vi "ONR Det Tube.vi"() -> ()   [LabVIEW 2018]
uses:
  <vilib>/Utility/file.llb/Write Delimited Spreadsheet (string).vi
  <vilib>/Analysis/NI_AALBase.lvlib
  <vilib>/Analysis/baseanly.llb/Mean (DBL).vi
  <vilib>/Utility/file.llb/Write Delimited Spreadsheet (DBL).vi
panel:
  out "Test row":string[](array[string])
  out "Test CSV Header":string[](array[string])
  out "vac err":dbl caption="Vacuum" format="%.3f %%"
  out "fuel err":dbl caption="Fuel" format="%.3f %%"
  out "ox err":dbl caption="Oxidizer" format="%.3f %%"
  out "dil err":dbl caption="Diluent" format="%.3f %%"
  in  "Vacuum Cutoff":dbl[unit]=689.4757889515781 format="%.2f"
  out "Fuel Cutoff":dbl[unit] caption="Fuel" format="%.2f"
  out "Oxidizer Cutoff":dbl[unit] caption="Oxidizer" format="%.2f"
  out "Diluent Cutoff":dbl[unit] caption="Diluent" format="%.2f"
  out "Test Status":string="No tests loaded"
  in  "Equivalence Ratio":string(combo)
  in  "Diluent":string(combo)
  in  "Diluent Mole Fraction":string(combo)
  in  "Fuel":string(combo)
  in  "Oxidizer":string(combo)
  in  "Initial Pressure":string(combo)
  out "indices":T1
  out "Test CSV":string[][](array[string])
  in  "Purge Time":dbl[unit] format="%#_13g"
  out "Remaining":dbl format="%<%M:%S>t"
  in  "Mix Time":dbl[unit]=180.0 format="%#_13g"
  out "Atmospheric (Calibrated)":dbl[unit]
  out "Diode read complete":bool
  out "Test Over?":bool
  in  "Tube valve delay (ms)":u32=4000
  out "Stop All":bool
  out "Stop Tests":bool
  in  "Pressure sample period (ms)":u32=100
  out "Record Diodes":bool
  out "Pressure Calibration":T2
  out "Pressure\nReadings":T3
  in  "Run Test":bool
  in  "Load Test CSV":bool
  in  "Current State":T4(ring)
  in  "Spark":bool
  in  "Mix Fan":bool
  in  "Stop Valve Control":bool
  in  "Atmospheric Pressure":dbl[unit] format="%.2f"
  in  "Valve Tube Inlet":bool
  in  "Valve Mix Inlet":bool
  in  "Valve Mix Outlet":bool
  in  "Valve Tube Outlet":bool=TRUE
  in  "Valve Oxidizer":bool
  in  "Valve Fuel":bool
  in  "Valve Diluent":bool
  in  "Valve Purge":bool
  in  "Valve Vacuum":bool
  in  "Set Mode":bool=TRUE
  out "Ambient Temp":dbl[unit]=567.411111111111 format="%.2f"
  out "Manifold Temp":dbl[unit]=294.2611111111111 format="%.2f"
  out "Tube Temp":dbl[unit]=294.2611111111111 format="%.2f"
  out "Manifold Pressure":dbl[unit] format="%.2f"
  out "Tube Pressure":dbl[unit] format="%.2f"
  out "System Pressures":T5(graph)={"Fuel Cutoff"=0.0, "Oxidizer Cutoff"=0.0, "Diluent Cutoff"=0.0, "Manifold Pressure"=-7310644.769423339, "Tube Pressure"=114564.88331091503}
  out "Completed fires":i32
  out "Pressure Unsafe?":bool
  # "Set Point"
  # "Error"
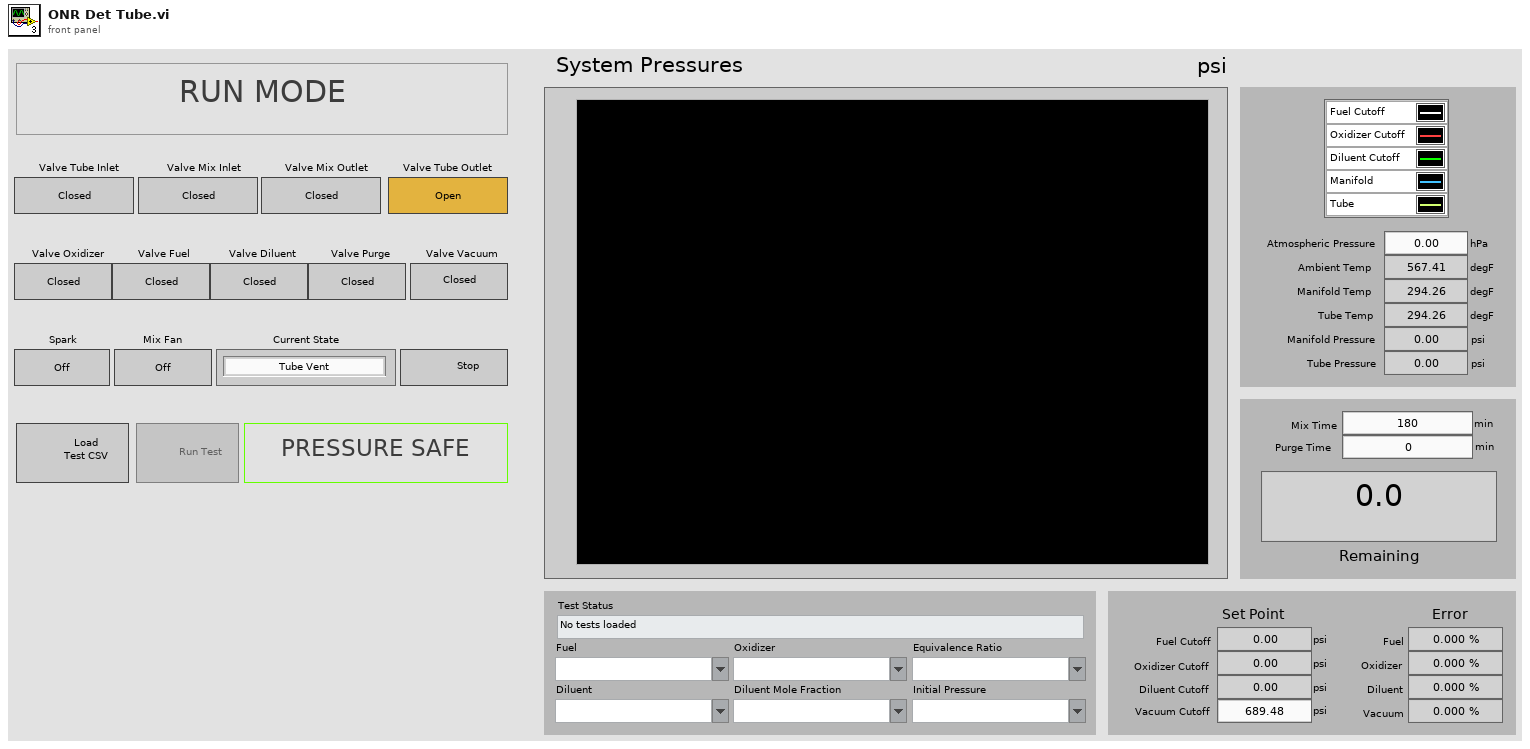
[diagram p1: front panel]
types:
  T1 = cluster{"fuel":i32, "oxidizer":i32, "diluent":i32, "diluent_mol_frac":i32, "equivalence":i32, "init_pressure":i32, "p_f":i32, "p_ox":i32, "p_dil":i32}
  T2 = cluster{"Manifold slope":dbl, "Manifold intercept":dbl, "Tube slope":dbl, "Tube intercept":dbl}
  T3 = cluster{"Time":timestamp, "Tube reading":dbl, "Manifold reading":dbl}
  T4 = enum16{"Tube Vent", "Mix Section Purge", "Tube Purge", "Tube Vacuum", "Diluent Fill", "Oxidizer Fill", "Fuel Fill", "Fill Hold", "Mixing", "Tube Closed", "Ignition", "Manifold Vent"}
  T5 = cluster{"Fuel Cutoff":dbl[unit], "Oxidizer Cutoff":dbl[unit], "Diluent Cutoff":dbl[unit], "Manifold Pressure":dbl[unit], "Tube Pressure":dbl[unit]}
  T6 = enum8{"Enabled", "Disabled", "Disabled and Grayed Out"}
  T7 = enum16{"open", "open or create", "create or replace", "create", "open (read-only)"}
  T8 = cluster{"Fuel Cutoff":dbl[unit], "Oxidizer Cutoff":dbl[unit], "Diluent Cutoff":dbl[unit], "Diluent Cutoff":dbl[unit], "Diluent Cutoff":dbl[unit]}[]
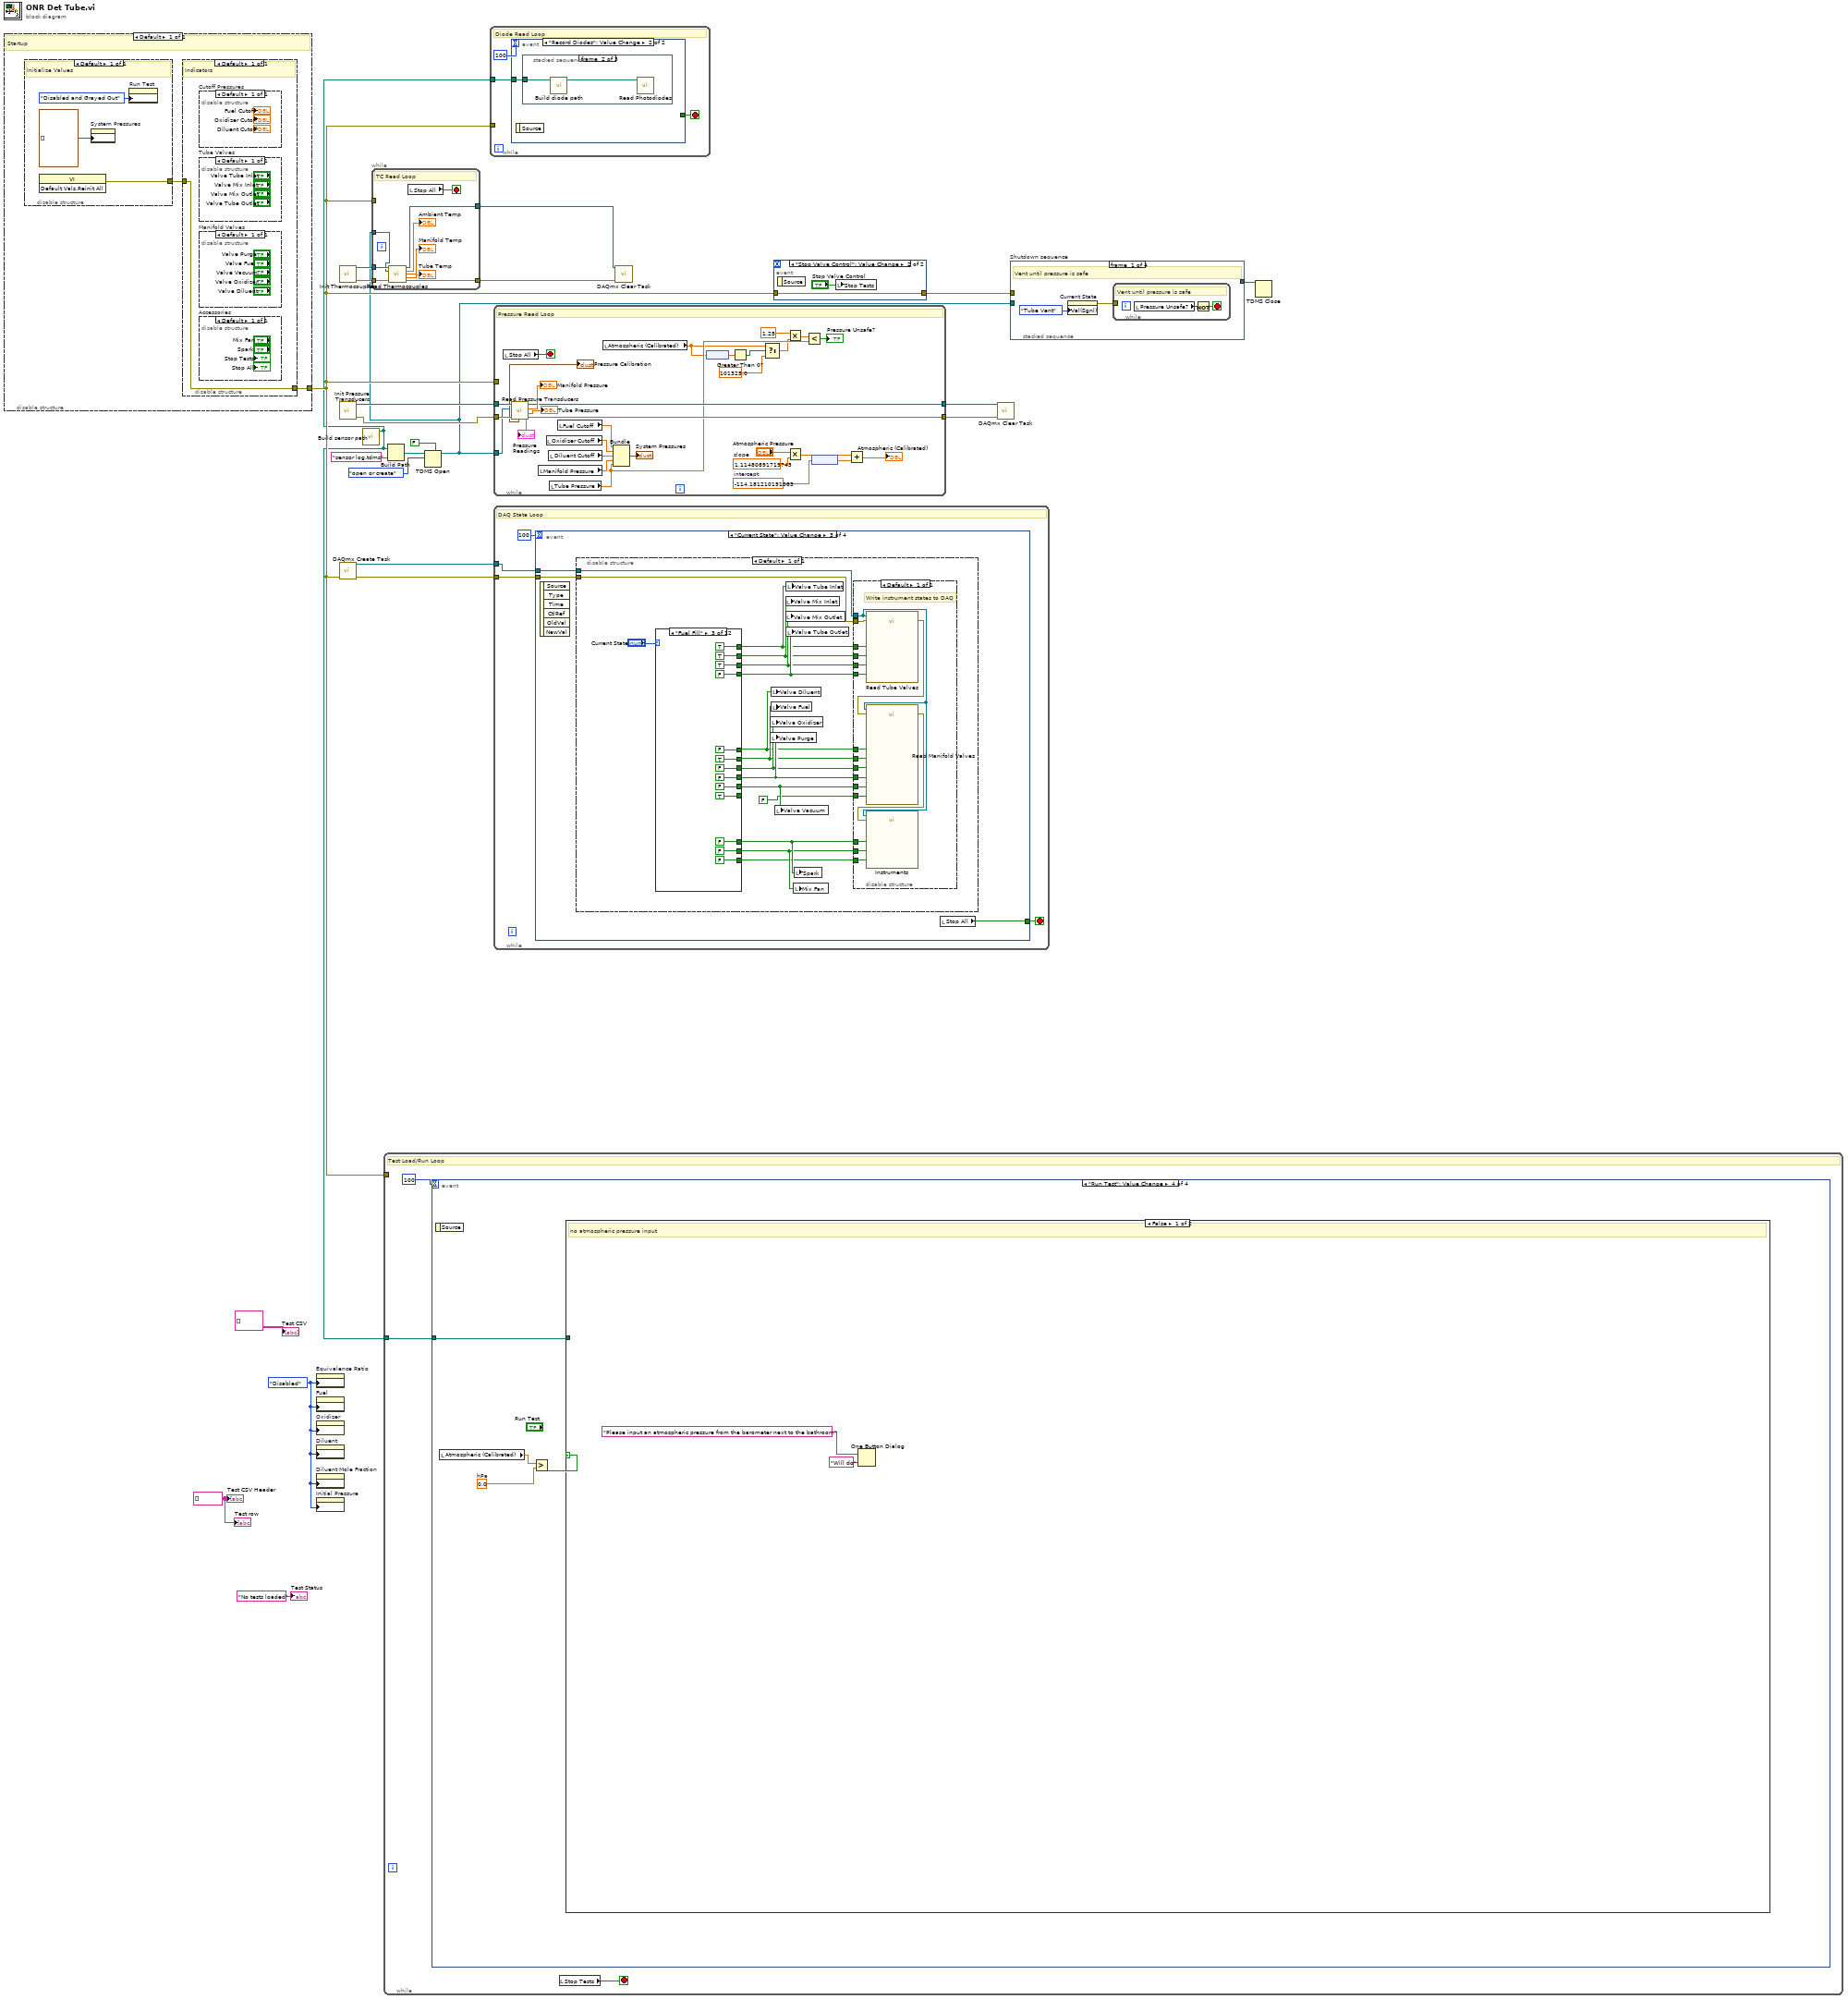
[diagram p0: block diagram]
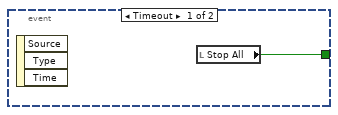
[diagram p2: hidden frame]
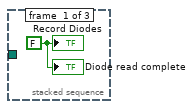
[diagram p3: hidden frame]
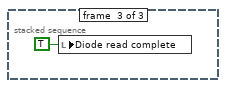
[diagram p4: hidden frame]
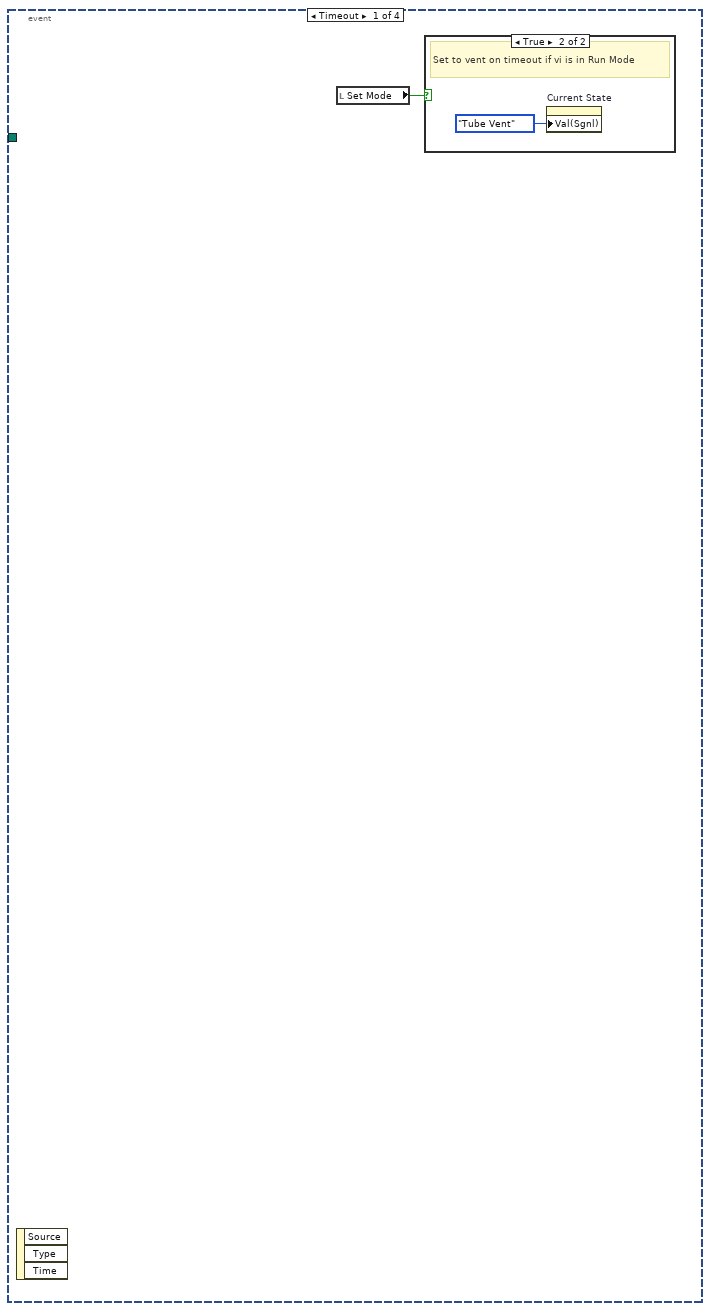
[diagram p5: hidden frame]
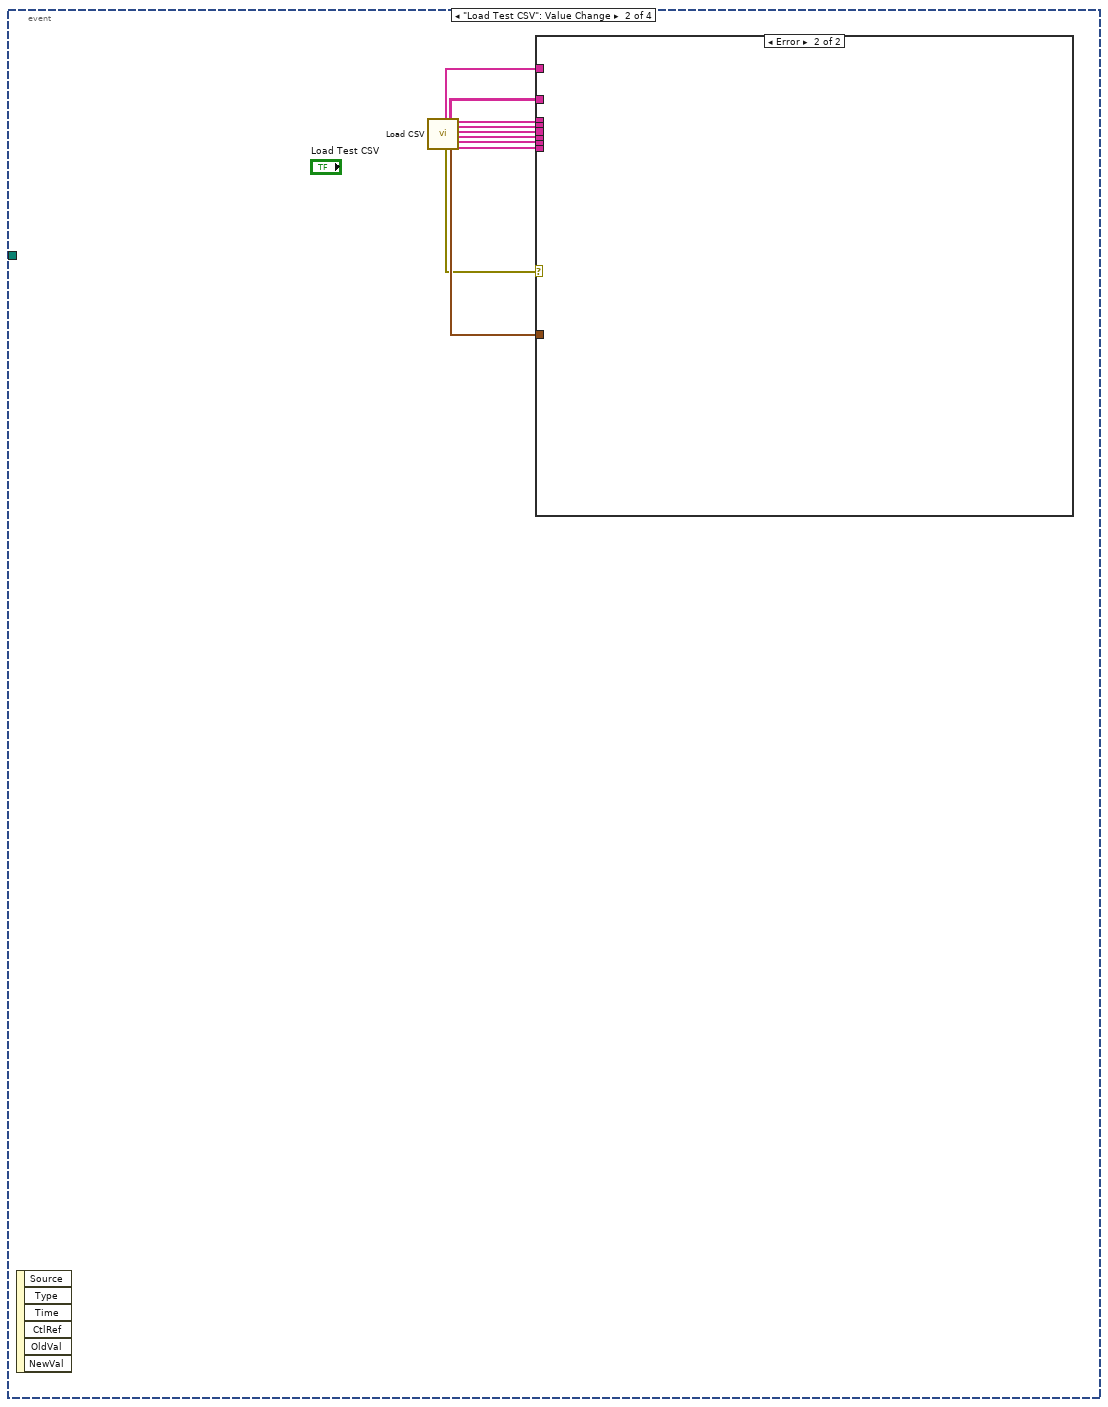
[diagram p7: hidden frame]
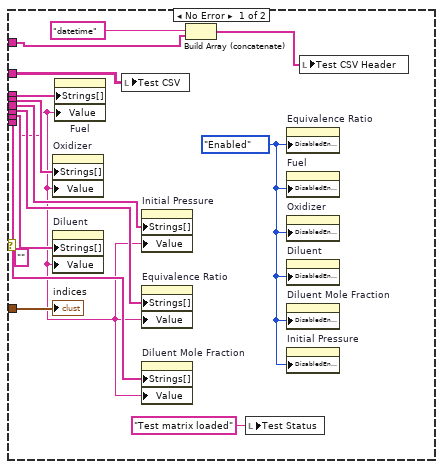
[diagram p8: hidden frame]
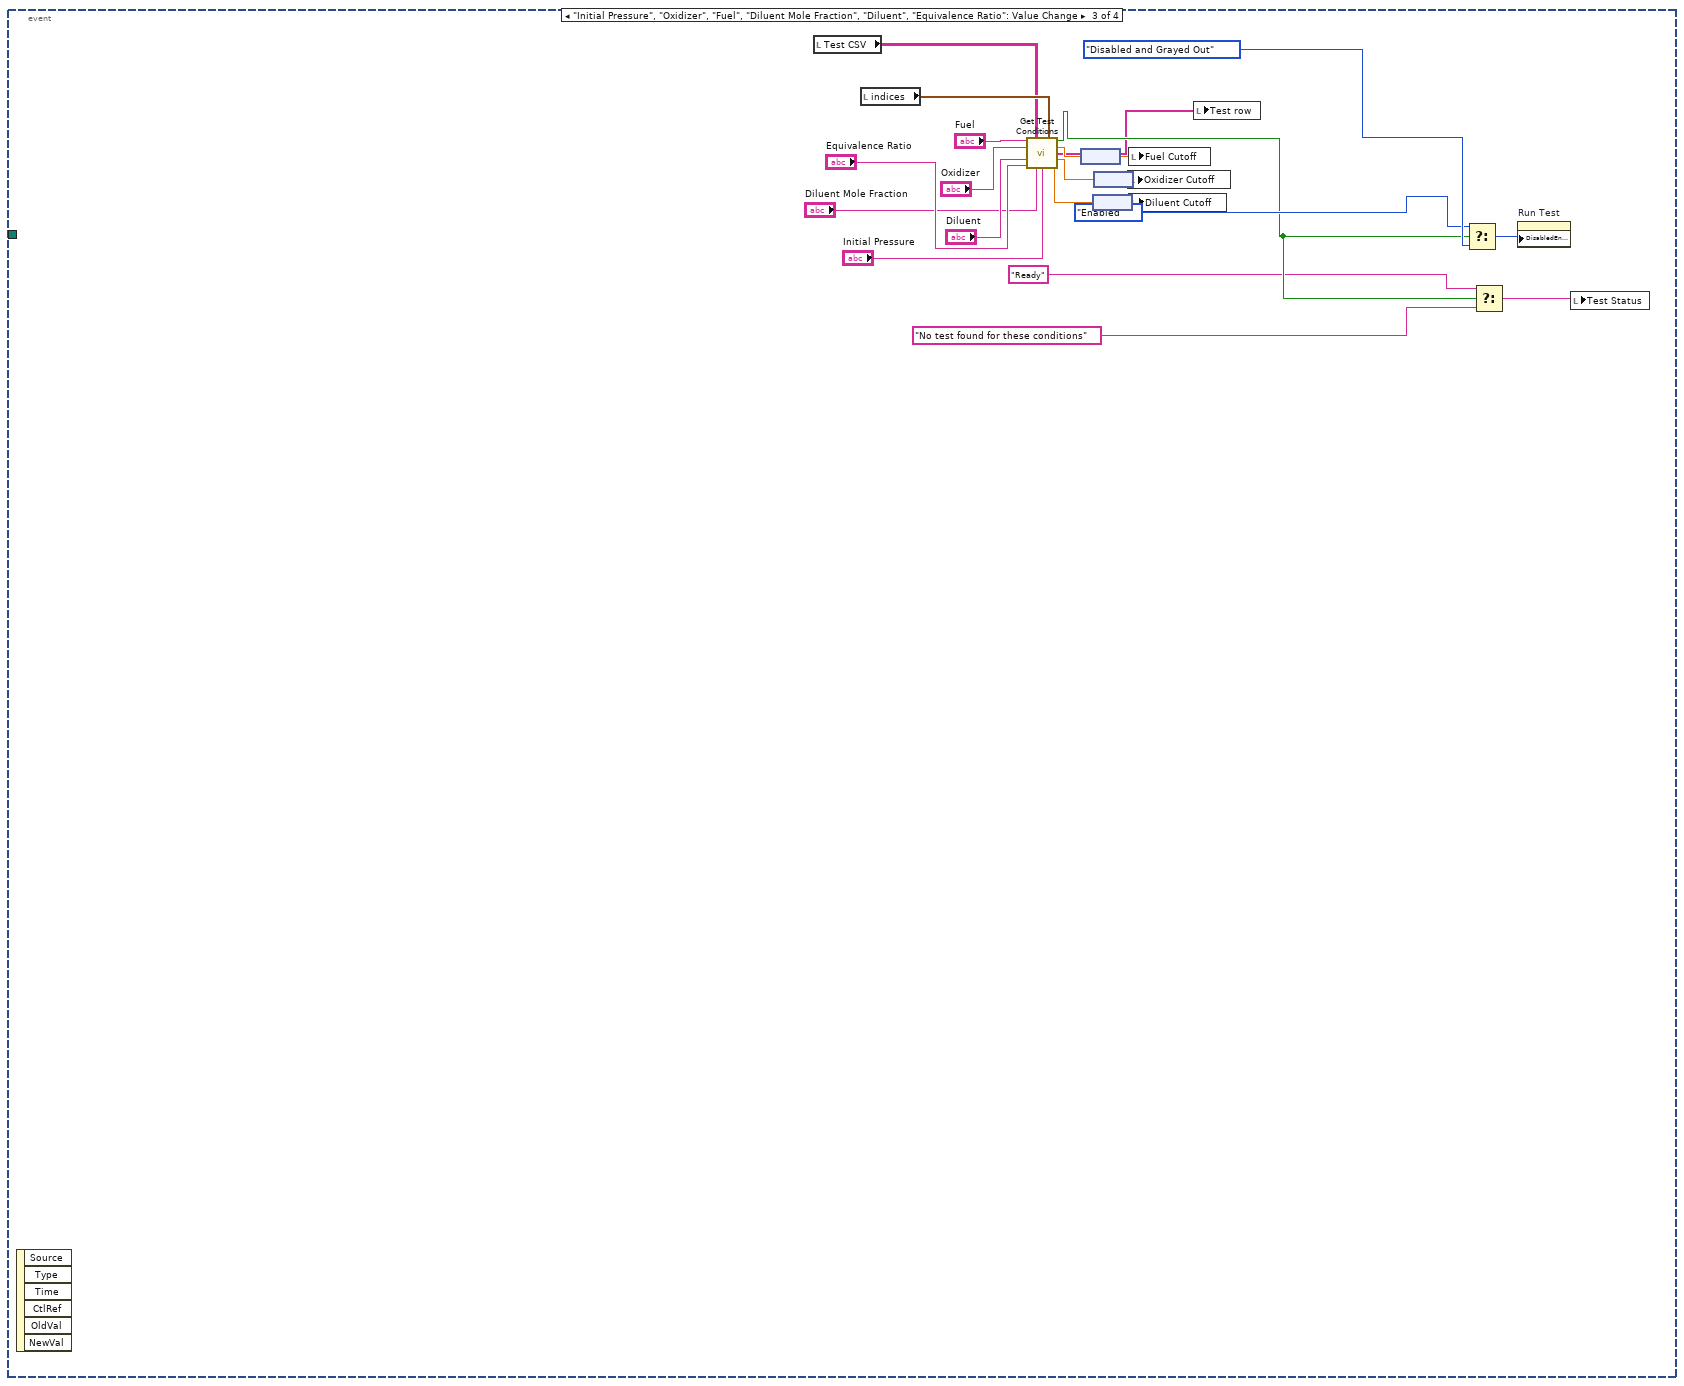
[diagram p9: hidden frame]
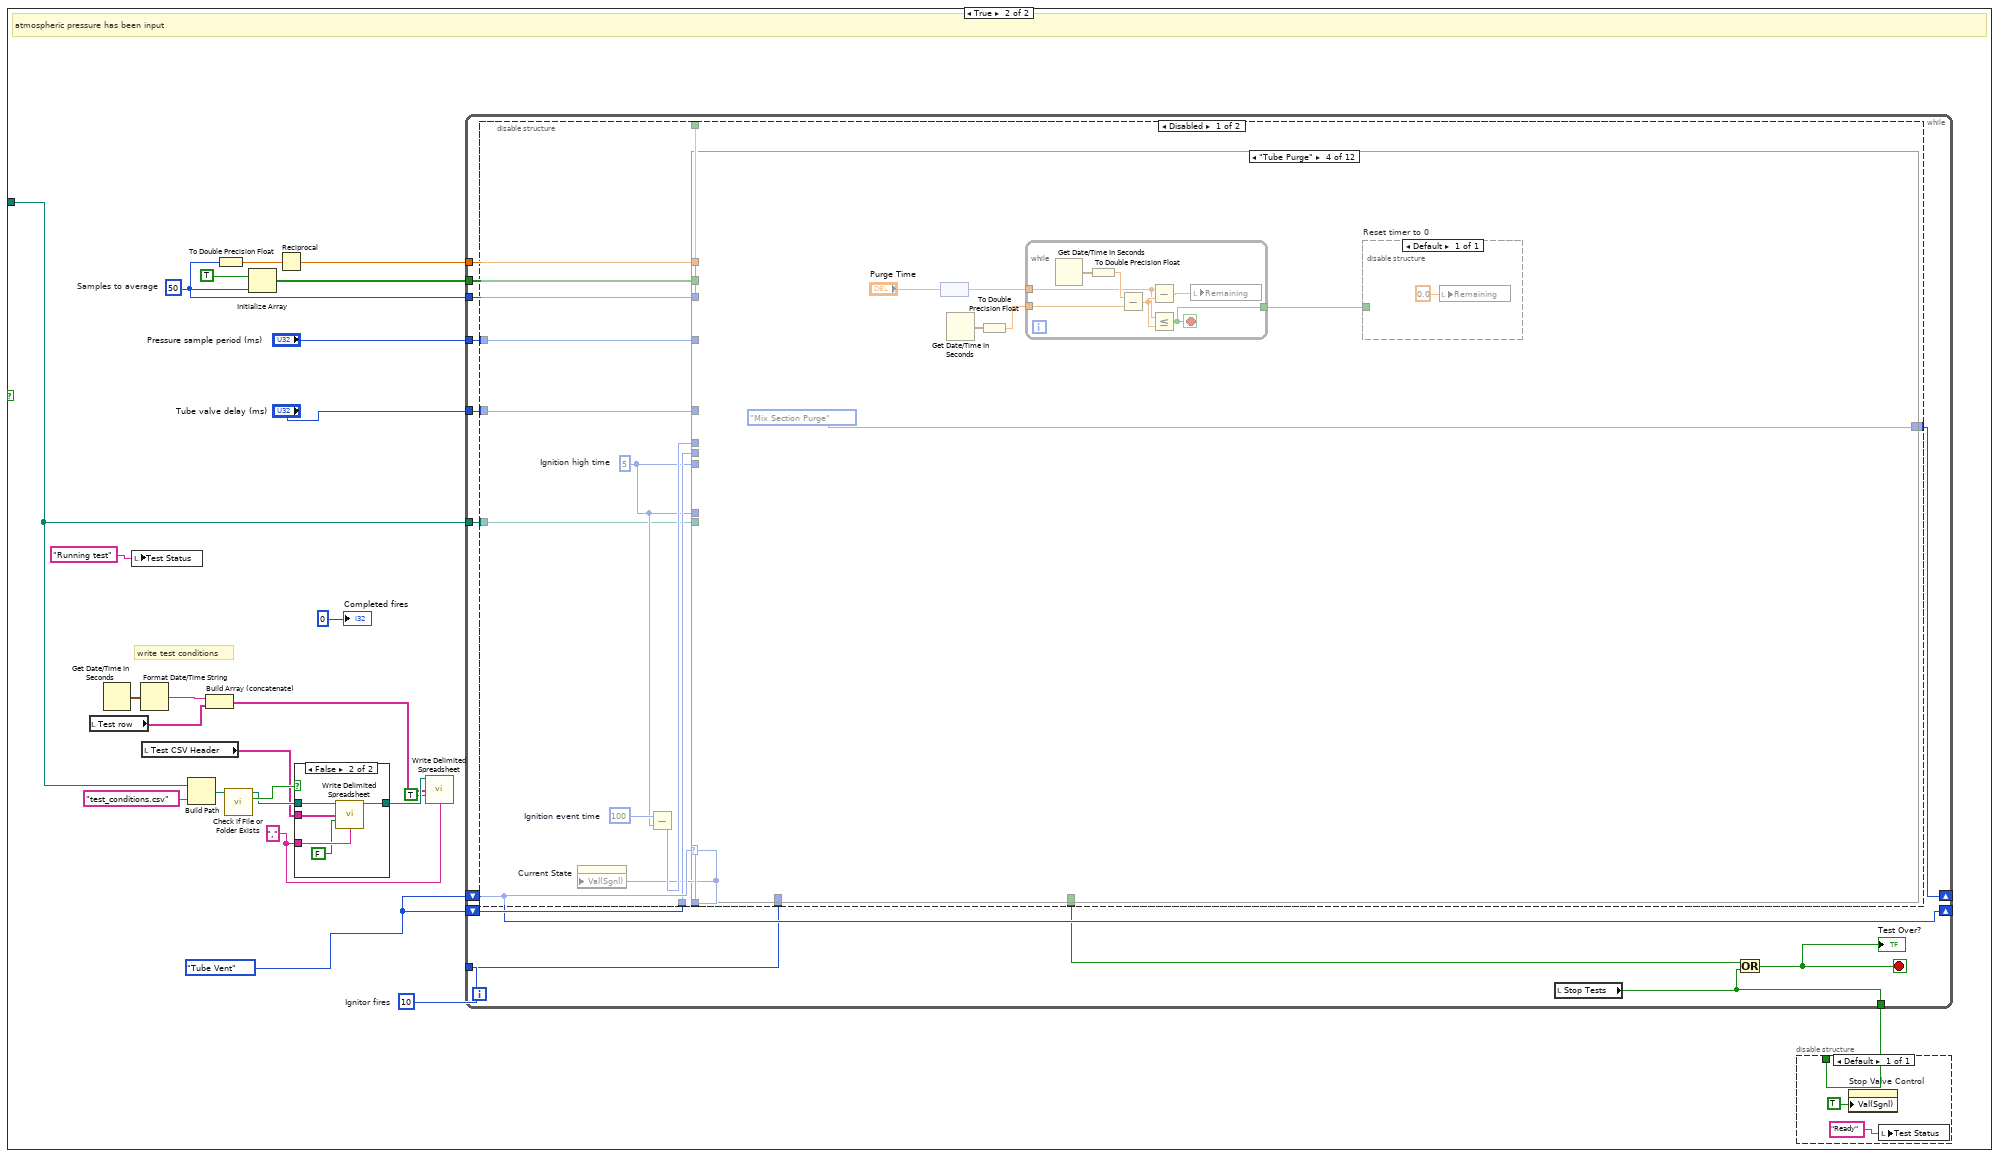
[diagram p10: hidden frame]
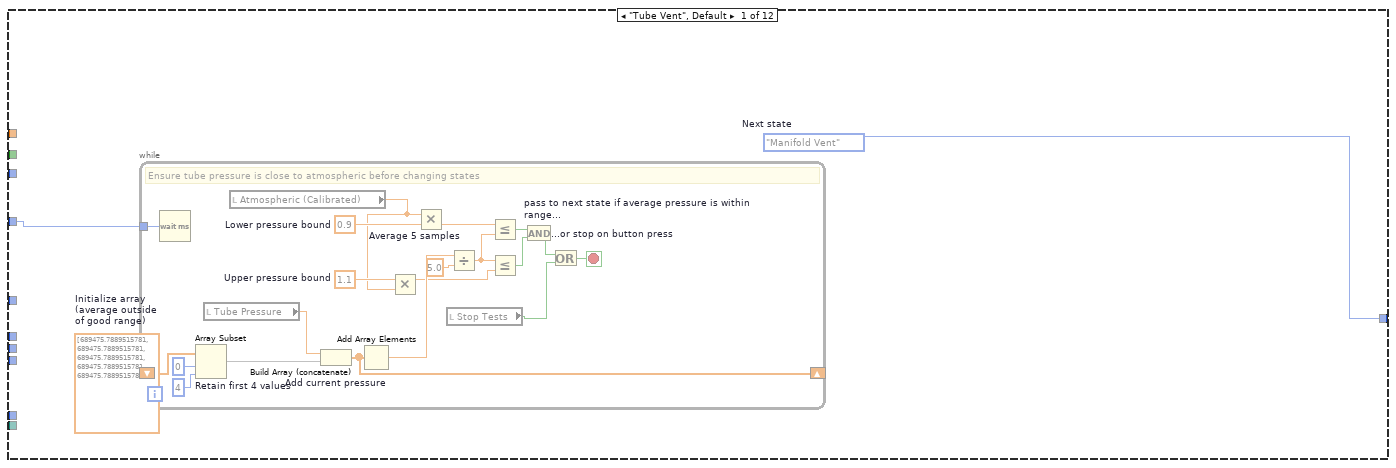
[diagram p12: hidden frame]
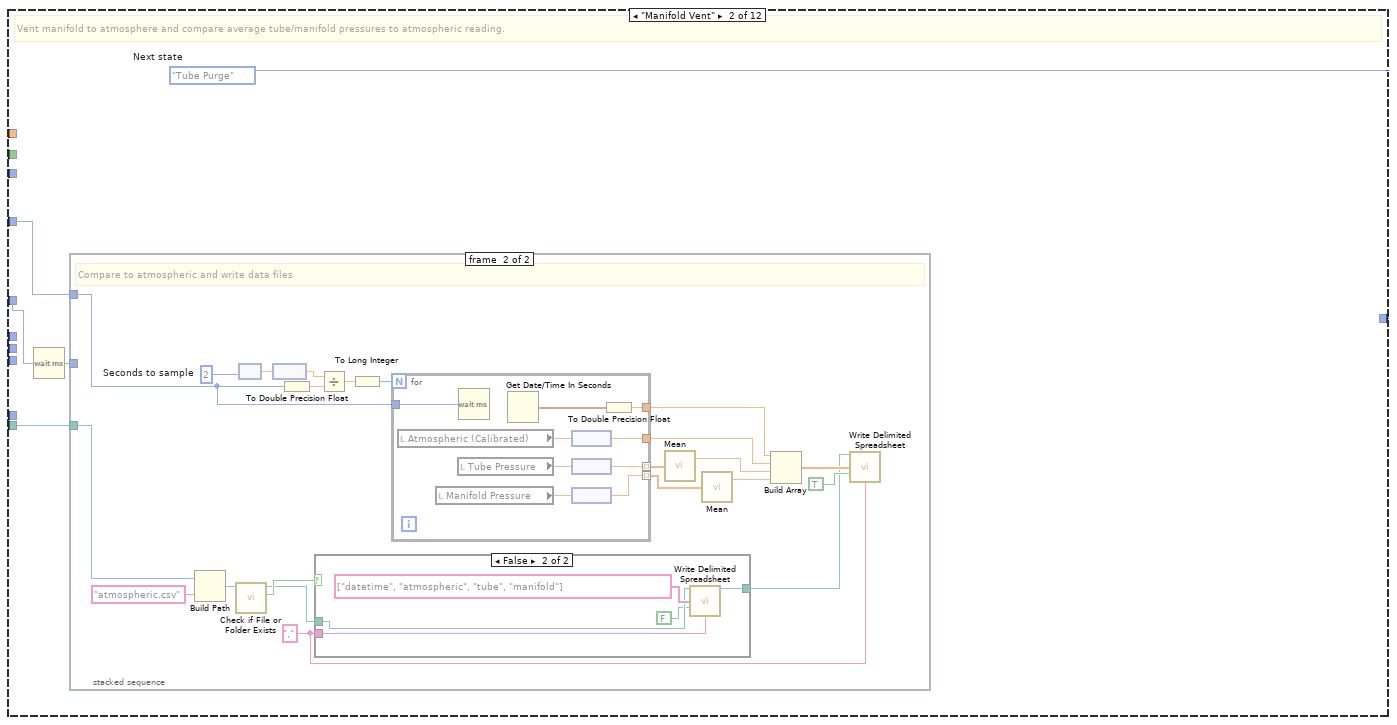
[diagram p13: hidden frame]
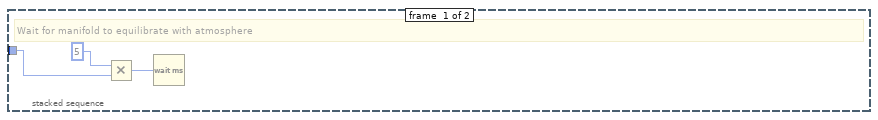
[diagram p14: hidden frame]
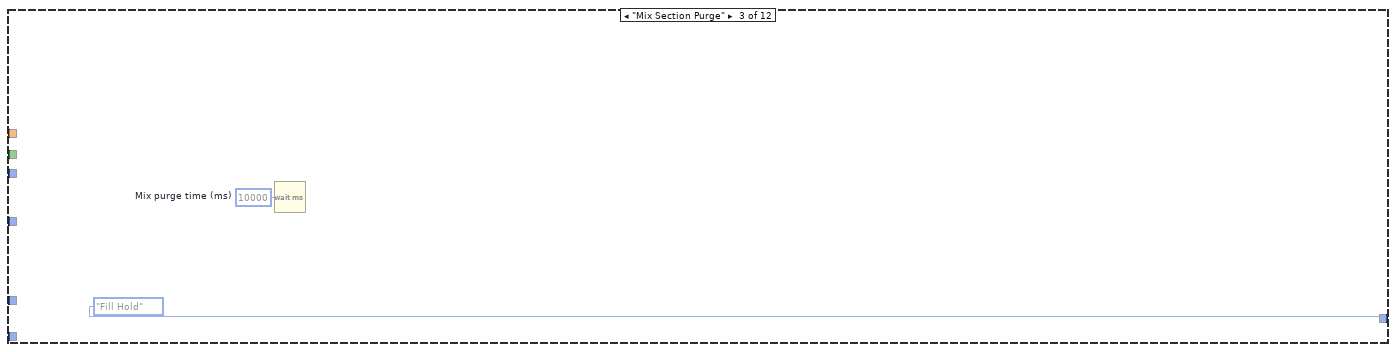
[diagram p16: hidden frame]
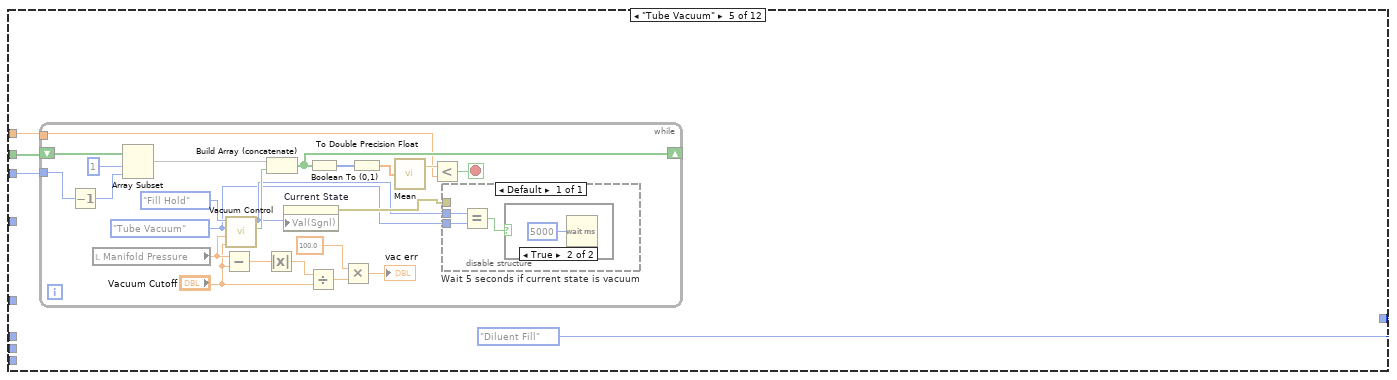
[diagram p17: hidden frame]
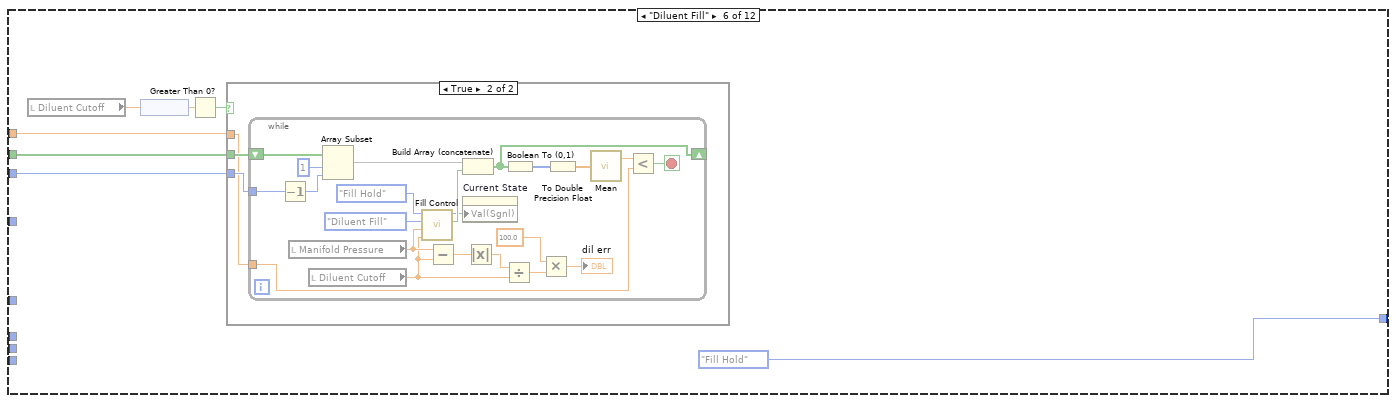
[diagram p19: hidden frame]
diagram:
  w1 = string[] []
  w2 = T6."Disabled" ("Disabled")
  n1 = disable-structure shown="Default" {
    disable-tunnel: [w24] -> w13
    frame Enabled {
      # "Startup"
      n2 = disable-structure shown="Default" {
        disable-tunnel: [w26] -> w25
        frame Enabled {
          # "Initialize Values"
          n3 = invoke class="VI" method="Default Vals.Reinit All"() -> (error out=w26:errorcluster)  [unwired: 3 in, 2 out]
          n4 = property on="System Pressures" class="WFChart (strict)"("History Data"=T8 []) -> ()  [unwired: 2 in, 2 out]
          n5 = property on="Run Test" class="Bool"("DisabledEnum"=T6."Disabled and Grayed Out" ("Disabled")) -> ()  [unwired: 2 in, 2 out]
        }
      }
      n6 = disable-structure shown="Default" {
        disable-tunnel: w25 -> [w29]
        disable-tunnel: [w29] -> w24
        frame Enabled {
          # "Indicators"
          n7 = disable-structure "Cutoff Pressures" shown="Default" {
            frame Enabled {
            }
          }
          n8 = disable-structure "Tube Valves" shown="Default" {
            frame Enabled {
            }
          }
          n9 = disable-structure "Manifold Valves" shown="Default" {
            frame Enabled {
            }
          }
          n10 = disable-structure "Accessories" shown="Default" {
            frame Enabled {
            }
          }
        }
      }
    }
  }
  n11 = property on="Equivalence Ratio" class="CmbBox"("DisabledEnum"=w2) -> ()  [unwired: 2 in, 2 out]
  n12 = property on="Fuel" class="CmbBox"("DisabledEnum"=w2) -> ()  [unwired: 2 in, 2 out]
  n13 = property on="Oxidizer" class="CmbBox"("DisabledEnum"=w2) -> ()  [unwired: 2 in, 2 out]
  n14 = property on="Diluent" class="CmbBox"("DisabledEnum"=w2) -> ()  [unwired: 2 in, 2 out]
  n15 = property on="Diluent Mole Fraction" class="CmbBox"("DisabledEnum"=w2) -> ()  [unwired: 2 in, 2 out]
  n16 = property on="Initial Pressure" class="CmbBox"("DisabledEnum"=w2) -> ()  [unwired: 2 in, 2 out]
  n17 = call "Init Thermocouples.vi"() -> ("task out"=w16:refnum<k21>, "Error Out"=w17:errorcluster)  [unwired: 14 in]
  n18 = call "Init Pressure Transducers.vi"() -> ("Error Out"=w21:errorcluster, "task out"=w20:refnum<k21>)  [unwired: 2 in]
  n19 = call <vilib>:"DAQmx Create Task.vi"("error in"=w13) -> ("task out"=w14:refnum<k21>, "error out"=w15:errorcluster)  [unwired: 13 in]
  n20 = call "Build sensor path.vi"() -> ("Current test directory"=w5:path)  [unwired: 9 in, 1 out]
  n21 = while {
    tunnel: w13 -> [_]
    tunnel: w5 -> [w30]
    stop <- w31 stop-if-true
    # "Test Load/Run Loop"
    n22 = event shown="[3] \"Run Test\": Value Change" {
      selector: _ -> [_ _ _ _]
      dyn-events: _ -> [_ _ _ _]
      timeout: 100 -> [_ _ _ _]
      tunnel: w30 -> [_ _ _ w81]
      event Timeout {
        n23 = event-data() -> ()  [unwired: 1 in, 3 out]
        n24 = local read "Set Mode"() -> (w33:bool)
        n25 = case shown="True" w33 {
          frame False {
          }
          frame True {
            # "Set to vent on timeout if vi is in Run Mode"
            n26 = property on="Current State" class="Enum (strict)"("Val(Sgnl)"=T4."Tube Vent" ("Current State 2")) -> ()  [unwired: 2 in, 2 out]
          }
        }
      }
      event "Load Test CSV": Value Change {
        n27 = event-data() -> ()  [unwired: 1 in, 6 out]
        n28 = call "Load CSV.vi"() -> ("Header"=w35:string[], "error out"=w36:errorcluster, "CSV Array"=w37:string[][], "indices"=w38:T1, "Fuel"=w41:string[], "Oxidizer"=w40:string[], "Initial Pressure"=w39:string[], "Equivalence Ratio"=w42:string[], "Diluent"=w43:string[], "Diluent Mole Fraction"=w44:string[])  [unwired: 10 in]
        n29 = case shown="Error" w36 {
          tunnel: w44 -> [w58 _]
          tunnel: w43 -> [w57 _]
          tunnel: w42 -> [w56 _]
          tunnel: w41 -> [w55 _]
          tunnel: w40 -> [w54 _]
          tunnel: w39 -> [w53 _]
          tunnel: w38 -> [w52 _]
          tunnel: w37 -> [w50 _]
          tunnel: w35 -> [w46 _]
          frame No Error {
            w48 = T6."Enabled" ("Disabled")
            w51 = "" ("Value (Signaling)")
            n30 = property on="Oxidizer" class="CmbBox"("Strings[]"=w54, "Value"=w51) -> ()  [unwired: 2 in, 2 out]
            n31 = property on="Diluent" class="CmbBox"("Strings[]"=w57, "Value"=w51) -> ()  [unwired: 2 in, 2 out]
            n32 = property on="Fuel" class="CmbBox"("Strings[]"=w55, "Value"=w51) -> ()  [unwired: 2 in, 2 out]
            n33 = local write "Test CSV"(w50) -> ()
            n34 = property on="Initial Pressure" class="CmbBox"("Strings[]"=w53, "Value"=w51) -> ()  [unwired: 2 in, 2 out]
            n35 = property on="Equivalence Ratio" class="CmbBox"("Strings[]"=w56, "Value"=w51) -> ()  [unwired: 2 in, 2 out]
            n36 = property on="Diluent Mole Fraction" class="CmbBox"("Strings[]"=w58, "Value"=w51) -> ()  [unwired: 2 in, 2 out]
            n37 = Build Array (concatenate)("datetime", w46) -> (w45:string[])
            n38 = local write "Test Status"("Test matrix loaded" ("Test Status")) -> ()
            n39 = property on="Equivalence Ratio" class="CmbBox"("DisabledEnum"=w48) -> ()  [unwired: 2 in, 2 out]
            n40 = property on="Fuel" class="CmbBox"("DisabledEnum"=w48) -> ()  [unwired: 2 in, 2 out]
            n41 = property on="Oxidizer" class="CmbBox"("DisabledEnum"=w48) -> ()  [unwired: 2 in, 2 out]
            n42 = property on="Diluent" class="CmbBox"("DisabledEnum"=w48) -> ()  [unwired: 2 in, 2 out]
            n43 = property on="Diluent Mole Fraction" class="CmbBox"("DisabledEnum"=w48) -> ()  [unwired: 2 in, 2 out]
            n44 = property on="Initial Pressure" class="CmbBox"("DisabledEnum"=w48) -> ()  [unwired: 2 in, 2 out]
            n45 = local write "Test CSV Header"(w45) -> ()
            "indices" <- w52
          }
          frame Error {
          }
        }
      }
      event "Initial Pressure", "Oxidizer", "Fuel", "Diluent Mole Fraction", "Diluent", "Equivalence Ratio": Value Change {
        n46 = event-data() -> ()  [unwired: 1 in, 6 out]
        n47 = local read "Test CSV"() -> (w67:string[][])
        n48 = local read "indices"() -> (w74:T1)
        n49 = call "Get Test Conditions.vi"("Fuel"="Fuel", "CSV Array"=w67, "indices"=w74, "Oxidizer"="Oxidizer", "Diluent"="Diluent", "Equivalence Ratio"="Equivalence Ratio", "Diluent Mole Fraction"="Diluent Mole Fraction", "Initial Pressure"="Initial Pressure") -> ("Test Found"=w63:bool, "Fuel Partial Pressure"=w73:dbl, "Test row"=w59:string[], "Oxidizer Partial Pressure"=w72:dbl, "Diluent Partial Pressure"=w71:dbl)  [unwired: 3 in]
        n50 = node(w73) -> (w70:dbl[unit])
        n51 = node(w71) -> (w68:dbl[unit])
        n52 = node(w72) -> (w69:dbl[unit])
        n53 = local write "Oxidizer Cutoff"(w69) -> ()
        n54 = local write "Fuel Cutoff"(w70) -> ()
        n55 = local write "Diluent Cutoff"(w68) -> ()
        n56 = local write "Test row"(w59) -> ()
        n57 = Select(t=T6."Enabled" ("Disabled"), s=w63, f=T6."Disabled and Grayed Out" ("Disabled")) -> (s? t:f=w66:T6)
        n58 = Select(t="Ready", s=w63, f="No test found for these conditions") -> (s? t:f=w62:string)
        n59 = property on="Run Test" class="Bool"("DisabledEnum"=w66) -> ()  [unwired: 2 in, 2 out]
        n60 = local write "Test Status"(w62) -> ()
      }
      event "Run Test": Value Change {
        w83 = dbl[unit] 0.0  # hPa
        n61 = event-data() -> ()  [unwired: 1 in, 1 out]
        n62 = local read "Atmospheric (Calibrated)"() -> (w84:dbl[unit])
        n63 = Greater?(x=w84, y=w83) -> (0:w82:bool)
        n64 = case shown="False" w82 {
          tunnel: w81 -> [_ w93]
          frame False {
            # "no atmospheric pressure input"
            n65 = One Button Dialog(message="Please input an atmospheric pressure from the barometer next to the bathroom" ("source"), button name ("OK")="Will do") -> ()  [unwired: 1 out]
          }
          frame True {
            w88 = "," ("delimiter (\\t)")
            w102 = 10  # Ignitor fires
            w104 = 50  # Samples to average
            w106 = T4."Tube Vent" ("Current State 2")
            # "write test conditions"
            # "atmospheric pressure has been input"
            n66 = local read "Test row"() -> (w90:string[])
            n67 = Get Date/Time In Seconds() -> (seconds since 1Jan1904=w99:timestamp)
            n68 = local write "Test Status"("Running test" ("Test Status")) -> ()
            n69 = Format Date/Time String(seconds (now)=w99) -> (date/time string=w98:string)  [unwired: 2 in]
            n70 = local read "Test CSV Header"() -> (w92:string[])
            n71 = Build Path(base path=w93, name or relative path="test_conditions.csv") -> (appended path=w95:path)
            n72 = Build Array (concatenate)(w98, w90) -> (w89:string[])
            n73 = To Double Precision Float(number=w104) -> (double precision float=w107:dbl)
            n74 = call <vilib>:"Check if File or Folder Exists.vi"("path"=w95) -> ("file or folder exists?"=w97:bool, "dup path"=w96:path)  [unwired: 8 in, 1 out]
            n75 = Initialize Array(TRUE, w104) -> (w109:bool[])
            n76 = Reciprocal(x=w107) -> (1/x=w110:dbl)
            n77 = case shown="False" w97 {
              tunnel: w88 -> [_ w117]
              tunnel: [w112 w116] -> w91
              tunnel: w96 -> [w112 w115]
              tunnel: w92 -> [_ w113]
              frame True {
              }
              frame False {
                n78 = call-poly <vilib>:"Write Delimited Spreadsheet.vi"("file path (dialog if empty)"=w115, "1D data"=w113, "append to file? (new file:F)"=FALSE, "delimiter (\\t)"=w117) -> ("new file path (Not A Path if cancelled)"=w116:path)  [unwired: 10 in, 1 out]
              }
            }
            n79 = call-poly <vilib>:"Write Delimited Spreadsheet.vi"("file path (dialog if empty)"=w91, "1D data"=w89, "append to file? (new file:F)"=TRUE, "delimiter (\\t)"=w88) -> ()  [unwired: 10 in, 2 out]
            n80 = while {
              shift-right: [w130] -> _
              shift-left: w106 -> [w123]
              shift-right: [w123] -> _
              shift-left: w106 -> [w129]
              tunnel: "Tube valve delay (ms)" -> [w127]
              tunnel: w109 -> [w124]
              tunnel: w104 -> [w125]
              tunnel: w110 -> [w126]
              tunnel: "Pressure sample period (ms)" -> [w128]
              tunnel: [w121] -> w103
              tunnel: w102 -> [w122]
              tunnel: w93 -> [w118]
              stop <- w120 stop-if-true
              n81 = disable-structure shown="Disabled" {
                disable-tunnel: [w144 _] -> w130
                disable-tunnel: w129 -> [w143 _]
                disable-tunnel: w128 -> [w142 _]
                disable-tunnel: w127 -> [w141 _]
                disable-tunnel: w126 -> [w140 _]
                disable-tunnel: w125 -> [w139 _]
                disable-tunnel: w124 -> [w138 _]
                disable-tunnel: w123 -> [w135 _]
                disable-tunnel: w122 -> [w134 _]
                disable-tunnel: [w133 _] -> w119
                disable-tunnel: w118 -> [w131 _]
                frame Disabled {
                  w137 = u32 100  # Ignition event time
                  w132 = u32 5  # Ignition high time
                  n82 = property on="Current State" class="Enum (strict)"("Val(Sgnl)"=w135) -> ()  [unwired: 2 in, 2 out]
                  n83 = Subtract(x=w137, y=w132) -> (x-y=w136:u32)
                  n84 = case shown="\"Tube Purge\"" w135 {
                    tunnel: [w147 w172 T4."Fill Hold" ("Current State 2") T4."Mix Section Purge" ("Current State 2") T4."Diluent Fill" ("Current State 2") T4."Fill Hold" ("Current State 2") T4."Fill Hold" ("Current State 2") T4."Fill Hold" ("Current State 2") w347 T4."Tube Closed" ("Current State 2") w378 T4."Tube Closed" ("Current State 2")] -> w144
                    tunnel: w143 -> [_ _ _ _ _ _ _ _ w348 _ w379 _]
                    tunnel: w142 -> [w146 w171 _ _ _ _ _ _ _ _ _ _]
                    tunnel: w141 -> [_ w170 _ _ _ _ _ _ w345 _ w376 _]
                    tunnel: w140 -> [_ _ _ _ w231 w261 w293 w320 _ _ _ _]
                    tunnel: w139 -> [_ _ _ _ w229 w263 w294 w319 _ _ _ _]
                    tunnel: w138 -> [_ _ _ _ w230 w262 w292 w318 _ _ _ _]
                    tunnel: w132 -> [_ _ _ _ _ _ _ _ _ _ _ _]
                    tunnel: w136 -> [_ _ _ _ _ _ _ _ _ _ w377 _]
                    tunnel: w134 -> [_ _ _ _ _ _ _ _ _ _ w375 _]
                    tunnel: [_ _ _ _ _ _ _ _ _ _ w374 _] -> w133
                    tunnel: w132 -> [_ _ _ _ _ _ _ _ _ _ _ w424]
                    tunnel: w131 -> [_ w168 _ _ _ _ _ _ _ _ w373 _]
                    frame "Tube Vent", Default {
                      w145 = dbl[unit][] [689475.7889515781, 689475.7889515781, 689475.7889515781, 689475.7889515781, 689475.7889515781]  # Initialize array (average outside of good range)
                      w147 = T4."Manifold Vent"  # Next state
                      n85 = while {
                        shift-right: [w166] -> _
                        shift-left: w145 -> [w165]
                        tunnel: w146 -> [w154]
                        stop <- w153 stop-if-true
                        w155 = 0.9  # Lower pressure bound
                        w159 = 1.1  # Upper pressure bound
                        # "Ensure tube pressure is close to atmospheric before changing states"
                        n86 = Wait (ms)(milliseconds to wait=w154) -> ()  [unwired: 1 out]
                        n87 = Array Subset "Retain first 4 values"(array=w165, index=0, length=4) -> (w161:dbl[unit][])
                        n88 = local read "Tube Pressure"() -> (w160:dbl[unit])
                        n89 = local read "Atmospheric (Calibrated)"() -> (w149:dbl[unit])
                        n90 = Build Array (concatenate) "Add current pressure"(w160, w161) -> (w166:dbl[unit][])
                        n91 = Add Array Elements(numeric array=w166) -> (sum=w167:dbl[unit])
                        n92 = Multiply(x=w159, y=w149) -> (x*y=w150:dbl[unit])
                        n93 = Multiply(x=w149, y=w155) -> (x*y=w151:dbl[unit])
                        n94 = local read "Stop Tests"() -> (w148:bool)
                        n95 = Divide "Average 5 samples"(x=w167, y=5.0 ("length")) -> (x/y=w156:dbl[unit])
                        n96 = Less Or Equal?(x=w151, y=w156) -> (x <= y?=w157:bool)
                        n97 = Less Or Equal?(x=w156, y=w150) -> (x <= y?=w158:bool)
                        n98 = And "pass to next state if average pressure is within range..."(x=w157, y=w158) -> (x .and. y?=w152:bool)
                        n99 = Or "...or stop on button press"(x=w152, y=w148) -> (x .or. y?=w153:bool)
                      }
                    }
                    frame "Manifold Vent" {
                      w172 = T4."Tube Purge"  # Next state
                      # "Vent manifold to atmosphere and compare average tube/manifold pressures to atmospheric reading."
                      n100 = Wait (ms)(milliseconds to wait=w170) -> (millisecond timer value=w169:u32)
                      n101 = stacked-sequence {
                        tunnel: w171 -> [w174 w197]
                        tunnel: w169 -> [_ _]
                        tunnel: w168 -> [_ w178]
                        frame #0 {
                          # "Wait for manifold to equilibrate with atmosphere"
                          n102 = Multiply(x=u32 5, y=w174) -> (x*y=w173:u32)
                          n103 = Wait (ms)(milliseconds to wait=w173) -> ()  [unwired: 1 out]
                        }
                        frame #1 {
                          w176 = "," ("delimiter (\\t)")
                          w195 = 2  # Seconds to sample
                          # "Compare to atmospheric and write data files"
                          n104 = Build Path(base path=w178, name or relative path="atmospheric.csv") -> (appended path=w180:path)
                          n105 = call <vilib>:"Check if File or Folder Exists.vi"("path"=w180) -> ("file or folder exists?"=w182:bool, "dup path"=w181:path)  [unwired: 8 in, 1 out]
                          n106 = node(w195) -> (w196:dbl[unit])
                          n107 = node(w196) -> (w194:dbl)
                          n108 = To Double Precision Float(number=w197) -> (double precision float=w191:dbl)
                          n109 = case shown="False" w182 {
                            tunnel: w176 -> [_ w203]
                            tunnel: [w198 w202] -> w183
                            tunnel: w181 -> [w198 w200]
                            frame True {
                            }
                            frame False {
                              n110 = call-poly <vilib>:"Write Delimited Spreadsheet.vi"("file path (dialog if empty)"=w200, "1D data"=string[] ["datetime", "atmospheric", "tube", "manifold"], "append to file? (new file:F)"=FALSE, "delimiter (\\t)"=w203) -> ("new file path (Not A Path if cancelled)"=w202:path)  [unwired: 10 in, 1 out]
                            }
                          }
                          n111 = Divide(x=w194, y=w191) -> (x/y=w193:dbl)
                          n112 = To Long Integer(number=w193) -> (32bit integer=w192:i32)
                          n113 = for {
                            N: w192 -> [_]
                            tunnel: w197 -> [w206]
                            tunnel: [w207] -> w189 mode=indexing
                            tunnel: [w208] -> w190 mode=indexing
                            tunnel: [w209] -> w186
                            tunnel: [w204] -> w177
                            n114 = local read "Atmospheric (Calibrated)"() -> (w210:dbl[unit])
                            n115 = local read "Manifold Pressure"() -> (w212:dbl[unit])
                            n116 = local read "Tube Pressure"() -> (w211:dbl[unit])
                            n117 = Wait (ms)(milliseconds to wait=w206) -> ()  [unwired: 1 out]
                            n118 = Get Date/Time In Seconds() -> (seconds since 1Jan1904=w205:timestamp)
                            n119 = node(w210) -> (w209:dbl)
                            n120 = node(w211) -> (w208:dbl)
                            n121 = node(w212) -> (w207:dbl)
                            n122 = To Double Precision Float(number=w205) -> (double precision float=w204:dbl)
                          }
                          n123 = call-poly <vilib>:"Mean.vi"("X"=w190) -> ("mean"=w187:dbl)  [unwired: 1 out]
                          n124 = call-poly <vilib>:"Mean.vi"("X"=w189) -> ("mean"=w188:dbl)  [unwired: 1 out]
                          n125 = Build Array(w177, w186, w187, w188) -> (w184:dbl[])
                          n126 = call-poly <vilib>:"Write Delimited Spreadsheet.vi"("file path (dialog if empty)"=w183, "1D data"=w184, "append to file? (new file:F)"=TRUE, "delimiter (\\t)"=w176) -> ()  [unwired: 10 in, 2 out]
                        }
                      }
                    }
                    frame "Mix Section Purge" {
                      w213 = u32 10000  # Mix purge time (ms)
                      n127 = Wait (ms)(milliseconds to wait=w213) -> ()  [unwired: 1 out]
                    }
                    frame "Tube Purge" {
                      n128 = node("Purge Time") -> (w215:dbl)
                      n129 = Get Date/Time In Seconds() -> (seconds since 1Jan1904=w218:timestamp)
                      n130 = To Double Precision Float(number=w218) -> (double precision float=w217:dbl)
                      n131 = while {
                        tunnel: w217 -> [w227]
                        tunnel: w215 -> [w224]
                        tunnel: [w223] -> w216
                        stop <- w223 stop-if-true
                        n132 = Get Date/Time In Seconds() -> (seconds since 1Jan1904=w228:timestamp)
                        n133 = To Double Precision Float(number=w228) -> (double precision float=w226:dbl)
                        n134 = Subtract(x=w226, y=w227) -> (x-y=w225:dbl)
                        n135 = Subtract(x=w224, y=w225) -> (x-y=w222:dbl)
                        n136 = Less Or Equal?(x=w224, y=w225) -> (x <= y?=w223:bool)
                        n137 = local write "Remaining"(w222) -> ()
                      }
                      n138 = disable-structure "Reset timer to 0" shown="Default" {
                        disable-tunnel: w216 -> [_]
                        frame Enabled {
                          n139 = local write "Remaining"(0.0 ("Remaining")) -> ()
                        }
                      }
                    }
                    frame "Tube Vacuum" {
                      n140 = while {
                        tunnel: w229 -> [w253]
                        shift-right: [w246] -> _
                        shift-left: w230 -> [w252]
                        tunnel: w231 -> [w245]
                        stop <- w244 stop-if-true
                        w233 = T4."Tube Vacuum" ("Current State 2")
                        n141 = Decrement(x=w253) -> (x-1=w255:i32)
                        n142 = local read "Manifold Pressure"() -> (w241:dbl[unit])
                        n143 = Array Subset(array=w252, index=1, length=w255) -> (w248:bool[])
                        n144 = Subtract(x=w241, y="Vacuum Cutoff") -> (x-y=w242:dbl[unit])
                        n145 = call "Vacuum Control.vi"("Fill Cutoff Pressure"="Vacuum Cutoff", "Manifold Pressure"=w241, "Fill State"=w233, "Hold State"=T4."Fill Hold" ("Current State 2")) -> ("Valve Open?"=w247:bool, "Output State"=w235:T4)  [unwired: 6 in]
                        n146 = Absolute Value(x=w242) -> (abs(x)=w243:dbl[unit])
                        n147 = Build Array (concatenate)(w248, w247) -> (w246:bool[])
                        n148 = property on="Current State" class="Enum (strict)"("Val(Sgnl)"=w235) -> (error out=w236:errorcluster)  [unwired: 2 in, 1 out]
                        n149 = Divide(x=w243, y="Vacuum Cutoff") -> (x/y=w240:dbl)
                        n150 = Boolean To (0,1)(Boolean=w246) -> (0, 1=w249:i16[])
                        n151 = Multiply(x=100.0, y=w240) -> (x*y=→"vac err":dbl)
                        n152 = To Double Precision Float(number=w249) -> (double precision float=w250:dbl[])
                        n153 = call-poly <vilib>:"Mean.vi"("X"=w250) -> ("mean"=w251:dbl)  [unwired: 1 out]
                        n154 = Less?(x=w251, y=w245) -> (x < y?=w244:bool)
                        n155 = disable-structure "Wait 5 seconds if current state is vacuum" shown="Default" {
                          disable-tunnel: w236 -> [_]
                          disable-tunnel: w235 -> [w257]
                          disable-tunnel: w233 -> [w256]
                          frame Enabled {
                            n156 = Equal?(x=w257, y=w256) -> (x = y?=w258:bool)
                            n157 = case shown="True" w258 {
                              frame False {
                              }
                              frame True {
                                n158 = Wait (ms)(milliseconds to wait=u32 5000) -> ()  [unwired: 1 out]
                              }
                            }
                          }
                        }
                      }
                    }
                    frame "Diluent Fill" {
                      n159 = local read "Diluent Cutoff"() -> (w264:dbl[unit])
                      n160 = node(w264) -> (w260:dbl)
                      n161 = Greater Than 0?(x=w260) -> (x > 0?=w265:bool)
                      n162 = case shown="True" w265 {
                        tunnel: w262 -> [_ w269]
                        tunnel: w263 -> [_ w268]
                        tunnel: w261 -> [_ w267]
                        frame False {
                        }
                        frame True {
                          n163 = while {
                            tunnel: w268 -> [w289]
                            shift-right: [w282] -> _
                            shift-left: w269 -> [w288]
                            tunnel: w267 -> [w281]
                            stop <- w280 stop-if-true
                            n164 = Decrement(x=w289) -> (x-1=w291:i32)
                            n165 = local read "Manifold Pressure"() -> (w277:dbl[unit])
                            n166 = local read "Diluent Cutoff"() -> (w276:dbl[unit])
                            n167 = Array Subset(array=w288, index=1, length=w291) -> (w284:bool[])
                            n168 = call "Fill Control.vi"("Fill Cutoff Pressure"=w276, "Manifold Pressure"=w277, "Fill State"=T4."Diluent Fill" ("Current State 2"), "Hold State"=T4."Fill Hold" ("Current State 2")) -> ("Valve Open?"=w283:bool, "Output State"=w273:T4)  [unwired: 6 in]
                            n169 = Subtract(x=w277, y=w276) -> (x-y=w278:dbl[unit])
                            n170 = Build Array (concatenate)(w284, w283) -> (w282:bool[])
                            n171 = property on="Current State" class="Enum (strict)"("Val(Sgnl)"=w273) -> ()  [unwired: 2 in, 2 out]
                            n172 = Absolute Value(x=w278) -> (abs(x)=w279:dbl[unit])
                            n173 = Divide(x=w279, y=w276) -> (x/y=w272:dbl)
                            n174 = Boolean To (0,1)(Boolean=w282) -> (0, 1=w285:i16[])
                            n175 = Multiply(x=100.0, y=w272) -> (x*y=→"dil err":dbl)
                            n176 = To Double Precision Float(number=w285) -> (double precision float=w286:dbl[])
                            n177 = call-poly <vilib>:"Mean.vi"("X"=w286) -> ("mean"=w287:dbl)  [unwired: 1 out]
                            n178 = Less?(x=w287, y=w281) -> (x < y?=w280:bool)
                          }
                        }
                      }
                    }
                    frame "Oxidizer Fill" {
                      n179 = while {
                        tunnel: w294 -> [w315]
                        shift-right: [w308] -> _
                        shift-left: w292 -> [w314]
                        tunnel: w293 -> [w307]
                        stop <- w306 stop-if-true
                        n180 = Decrement(x=w315) -> (x-1=w317:i32)
                        n181 = local read "Manifold Pressure"() -> (w303:dbl[unit])
                        n182 = local read "Oxidizer Cutoff"() -> (w302:dbl[unit])
                        n183 = Array Subset(array=w314, index=1, length=w317) -> (w310:bool[])
                        n184 = Subtract(x=w303, y=w302) -> (x-y=w304:dbl[unit])
                        n185 = call "Fill Control.vi"("Fill Cutoff Pressure"=w302, "Manifold Pressure"=w303, "Fill State"=T4."Oxidizer Fill" ("Current State 2"), "Hold State"=T4."Fill Hold" ("Current State 2")) -> ("Valve Open?"=w309:bool, "Output State"=w299:T4)  [unwired: 6 in]
                        n186 = Absolute Value(x=w304) -> (abs(x)=w305:dbl[unit])
                        n187 = Build Array (concatenate)(w310, w309) -> (w308:bool[])
                        n188 = property on="Current State" class="Enum (strict)"("Val(Sgnl)"=w299) -> ()  [unwired: 2 in, 2 out]
                        n189 = Divide(x=w305, y=w302) -> (x/y=w298:dbl)
                        n190 = Boolean To (0,1)(Boolean=w308) -> (0, 1=w311:i16[])
                        n191 = Multiply(x=100.0, y=w298) -> (x*y=→"ox err":dbl)
                        n192 = To Double Precision Float(number=w311) -> (double precision float=w312:dbl[])
                        n193 = call-poly <vilib>:"Mean.vi"("X"=w312) -> ("mean"=w313:dbl)  [unwired: 1 out]
                        n194 = Less?(x=w313, y=w307) -> (x < y?=w306:bool)
                      }
                    }
                    frame "Fuel Fill" {
                      n195 = while {
                        tunnel: w319 -> [w341]
                        shift-right: [w334] -> _
                        shift-left: w318 -> [w340]
                        tunnel: w320 -> [w333]
                        stop <- w332 stop-if-true
                        n196 = Decrement(x=w341) -> (x-1=w343:i32)
                        n197 = local read "Manifold Pressure"() -> (w329:dbl[unit])
                        n198 = Array Subset(array=w340, index=1, length=w343) -> (w336:bool[])
                        n199 = local read "Fuel Cutoff"() -> (w328:dbl[unit])
                        n200 = Subtract(x=w329, y=w328) -> (x-y=w330:dbl[unit])
                        n201 = call "Fill Control.vi"("Fill Cutoff Pressure"=w328, "Manifold Pressure"=w329, "Fill State"=T4."Fuel Fill" ("Current State 2"), "Hold State"=T4."Fill Hold" ("Current State 2")) -> ("Valve Open?"=w335:bool, "Output State"=w325:T4)  [unwired: 6 in]
                        n202 = Absolute Value(x=w330) -> (abs(x)=w331:dbl[unit])
                        n203 = Build Array (concatenate)(w336, w335) -> (w334:bool[])
                        n204 = property on="Current State" class="Enum (strict)"("Val(Sgnl)"=w325) -> ()  [unwired: 2 in, 2 out]
                        n205 = Divide(x=w331, y=w328) -> (x/y=w323:dbl)
                        n206 = Boolean To (0,1)(Boolean=w334) -> (0, 1=w337:i16[])
                        n207 = Multiply(x=100.0, y=w323) -> (x*y=→"fuel err":dbl)
                        n208 = To Double Precision Float(number=w337) -> (double precision float=w338:dbl[])
                        n209 = call-poly <vilib>:"Mean.vi"("X"=w338) -> ("mean"=w339:dbl)  [unwired: 1 out]
                        n210 = Less?(x=w339, y=w333) -> (x < y?=w332:bool)
                      }
                    }
                    frame "Fill Hold" {
                      w346 = u32 2000  # Fill hold time (ms)
                      # "All manifold valves are shut off, while the tube is left open to the manifold so that the pressure can equalize. Next state is decided by the previous state."
                      n211 = Get Date/Time In Seconds() -> (seconds since 1Jan1904=w344:timestamp)
                      n212 = To Double Precision Float(number=w344) -> ()  [unwired: 1 out]
                      n213 = case "Decide course of action based on previous state" shown="\"Oxidizer Fill\"" w348 {
                        tunnel: [T4."Oxidizer Fill" ("Current State 2") T4."Fuel Fill" ("Current State 2") T4."Tube Vacuum" ("Current State 2") T4."Tube Vent" ("Current State 2") T4."Tube Closed" ("Current State 2")] -> w347
                        tunnel: w346 -> [w349 w351 _ w355 w357]
                        tunnel: w345 -> [_ _ w353 _ _]
                        frame "Diluent Fill" {
                          n214 = Wait (ms)(milliseconds to wait=w349) -> ()  [unwired: 1 out]
                        }
                        frame "Oxidizer Fill" {
                          n215 = Wait (ms)(milliseconds to wait=w351) -> ()  [unwired: 1 out]
                        }
                        frame "Mix Section Purge" {
                          n216 = Wait (ms)(milliseconds to wait=w353) -> ()  [unwired: 1 out]
                        }
                        frame "Tube Vent", Default {
                          n217 = Wait (ms)(milliseconds to wait=w355) -> ()  [unwired: 1 out]
                        }
                        frame "Fuel Fill" {
                          n218 = Wait (ms)(milliseconds to wait=w357) -> ()  [unwired: 1 out]
                        }
                      }
                    }
                    frame "Mixing" {
                      n219 = Get Date/Time In Seconds() -> (seconds since 1Jan1904=w363:timestamp)
                      n220 = To Double Precision Float(number=w363) -> (double precision float=w362:dbl)
                      n221 = node("Mix Time") -> (w360:dbl)
                      n222 = while {
                        tunnel: w362 -> [w371]
                        tunnel: w360 -> [w367]
                        tunnel: [w366] -> w359
                        stop <- w366 stop-if-true
                        n223 = Get Date/Time In Seconds() -> (seconds since 1Jan1904=w372:timestamp)
                        n224 = To Double Precision Float(number=w372) -> (double precision float=w370:dbl)
                        n225 = Subtract(x=w370, y=w371) -> (x-y=w368:dbl)
                        n226 = Subtract(x=w367, y=w368) -> (x-y=→"Remaining":dbl)
                        n227 = Less Or Equal?(x=w367, y=w368) -> (x <= y?=w366:bool)
                      }
                      n228 = disable-structure "Reset timer to 0" shown="Default" {
                        disable-tunnel: w359 -> [_]
                        frame Enabled {
                          n229 = local write "Remaining"(0.0 ("Remaining")) -> ()
                        }
                      }
                    }
                    frame "Tube Closed" {
                      n230 = case shown="\"Ignition\"" w379 {
                        tunnel: [w386 T4."Mixing" ("Current State 2") w398 T4."Tube Vent" ("Current State 2")] -> w378
                        tunnel: w375 -> [_ _ w396 _]
                        tunnel: w377 -> [_ _ w394 _]
                        tunnel: w376 -> [w385 w392 _ _]
                        tunnel: [_ _ w395 _] -> w374
                        tunnel: w373 -> [w380 _ _ _]
                        frame "Mixing" {
                          n231 = Wait (ms)(milliseconds to wait=w385) -> (millisecond timer value=w384:u32)
                          n232 = disable-structure shown="Default" {
                            disable-tunnel: w384 -> [_]
                            disable-tunnel: [w390] -> w383
                            frame Enabled {
                              n233 = property on="Record Diodes" class="Bool (strict)"("Val(Sgnl)"=TRUE ("Spark")) -> (error out=w390:errorcluster)  [unwired: 2 in, 1 out]
                            }
                          }
                          n234 = disable-structure shown="Default" {
                            disable-tunnel: w383 -> [_]
                            disable-tunnel: [w387] -> w382
                            frame Enabled {
                              n235 = Wait (ms)(milliseconds to wait=u32 500) -> (millisecond timer value=w387:u32)
                            }
                          }
                          n236 = call "Write Ignition Time.vi"("file path"=w380) -> ("tdms file out"=w381:refnum<k34>)  [unwired: 1 in, 1 out]
                          n237 = disable-structure shown="Default" {
                            disable-tunnel: [T4."Ignition" ("Current State 2")] -> w386
                            disable-tunnel: w382 -> [_]
                            disable-tunnel: w381 -> [_]
                            frame Enabled {
                            }
                          }
                        }
                        frame "Fill Hold" {
                          n238 = Wait (ms)(milliseconds to wait=w392) -> ()  [unwired: 1 out]
                        }
                        frame "Ignition" {
                          n239 = local read "Completed fires"() -> (w397:i32)
                          n240 = Less?(x=w397, y=w396) -> (x < y?=w399:bool)
                          n241 = case shown="False" w399 {
                            tunnel: [w404 T4."Ignition" ("Current State 2")] -> w398
                            tunnel: w394 -> [_ _]
                            tunnel: [w403 _] -> w395
                            tunnel: w394 -> [_ w415]
                            frame False {
                              n242 = disable-structure shown="Default" {
                                disable-tunnel: [w405] -> w400
                                frame Enabled {
                                n243 = call <vilib>:"DAQmx Create Task.vi"("new task name"="spark", "error in"=errorcluster {"status"=FALSE, "code"=0, "source"=""}) -> ("task out"=w409:refnum<k21>, "error out"=w410:errorcluster)  [unwired: 12 in]
                                n244 = call "Instruments.vi"("task in"=w409, "Error In"=w410, "Spark"=FALSE) -> ("Error Out"=w405:errorcluster)  [unwired: 13 in, 3 out]
                                }
                              }
                              n245 = while {
                                tunnel: [w414] -> w403
                                tunnel: [w414] -> w401
                                tunnel: w400 -> [_]
                                stop <- w414 stop-if-true
                                n246 = local read "Diode read complete"() -> (w414:bool)
                              }
                              n247 = disable-structure shown="Default" {
                                disable-tunnel: [w412] -> w402
                                disable-tunnel: w401 -> [_]
                                frame Enabled {
                                # "...just wait longer"
                                n248 = Wait (ms)(milliseconds to wait=u32 5000) -> (millisecond timer value=w412:u32)
                                }
                              }
                              n249 = disable-structure shown="Default" {
                                disable-tunnel: [T4."Tube Vent" ("Current State 2")] -> w404
                                disable-tunnel: w402 -> [_]
                                frame Enabled {
                                }
                              }
                            }
                            frame True {
                              n250 = flat-sequence {
                                tunnel: w415 -> [w422]
                                frame #0 {
                                n251 = call <vilib>:"DAQmx Create Task.vi"("new task name"="spark", "error in"=errorcluster {"status"=FALSE, "code"=0, "source"=""}) -> ("task out"=w420:refnum<k21>, "error out"=w421:errorcluster)  [unwired: 12 in]
                                n252 = call "Instruments.vi"("task in"=w420, "Error In"=w421, "Spark"=FALSE) -> ()  [unwired: 13 in, 4 out]
                                }
                                frame #1 {
                                n253 = Wait (ms) "Ignition low time"(milliseconds to wait=w422) -> ()  [unwired: 1 out]
                                }
                              }
                            }
                          }
                        }
                        frame "Tube Vent", Default {
                          # "default case, please ignore"
                        }
                      }
                    }
                    frame "Ignition" {
                      n254 = flat-sequence {
                        tunnel: w424 -> [w431]
                        frame #0 {
                          n255 = call <vilib>:"DAQmx Create Task.vi"("new task name"="spark", "error in"=errorcluster {"status"=FALSE, "code"=0, "source"=""}) -> ("task out"=w429:refnum<k21>, "error out"=w430:errorcluster)  [unwired: 12 in]
                          n256 = call "Instruments.vi"("task in"=w429, "Error In"=w430, "Spark"=TRUE) -> ()  [unwired: 13 in, 4 out]
                        }
                        frame #1 {
                          n257 = Wait (ms)(milliseconds to wait=w431) -> ()  [unwired: 1 out]
                        }
                        frame #2 {
                          n258 = local read "Completed fires"() -> (w432:i32)
                          n259 = Increment(x=w432) -> (x+1=w433:i32)
                          n260 = local write "Completed fires"(w433) -> ()
                        }
                      }
                    }
                  }
                }
                frame Enabled {
                }
              }
              n261 = local read "Stop Tests"() -> (w121:bool)
              n262 = Or(x=w119, y=w121) -> (x .or. y?=w120:bool)
              "Test Over?" <- w120
            }
            n263 = disable-structure shown="Default" {
              disable-tunnel: w103 -> [_]
              frame Enabled {
                n264 = property on="Stop Valve Control" class="Bool (strict)"("Val(Sgnl)"=TRUE ("Value (Signaling)")) -> ()  [unwired: 2 in, 2 out]
                n265 = local write "Test Status"("Ready" ("Test Status")) -> ()
              }
            }
            "Completed fires" <- 0 ("Completed fires")
          }
        }
      }
    }
    n266 = local read "Stop Tests"() -> (w31:bool)
  }
  n267 = Build Path(base path=w5, name or relative path="sensor log.tdms") -> (appended path=w9:path)
  n268 = TDMS Open(5:FALSE ("create index file? (T)"), 10:T7."open or create" ("operation (0:open)"), 11:w9) -> (3:w7:refnum<k34>)  [unwired: 4 in, 1 out]
  n269 = while {
    tunnel: w16 -> [w441]
    tunnel: w17 -> [w440]
    tunnel: [w439] -> w18
    tunnel: [w438] -> w19
    tunnel: w13 -> [_]
    tunnel: w7 -> [w436]
    stop <- w437 stop-if-true
    # "TC Read Loop"
    n270 = call "Read Thermocouples.vi"("task in"=w441, "tdms file"=w436, "Error In"=w440) -> ("task out"=w439:refnum<k21>, "Ambient Temp"=→"Ambient Temp":dbl[unit], "Manifold Temp"=→"Manifold Temp":dbl[unit], "Tube Temp"=→"Tube Temp":dbl[unit], "Error Out"=w438:errorcluster)  [unwired: 8 in]
    n271 = local read "Stop All"() -> (w437:bool)
  }
  n272 = while {
    tunnel: w13 -> [_]
    tunnel: w5 -> [w445]
    stop <- w447 stop-if-true
    # "Diode Read Loop"
    n273 = event shown="[1] \"Record Diodes\": Value Change" {
      selector: _ -> [_ _]
      dyn-events: _ -> [_ _]
      timeout: 100 -> [_ _]
      tunnel: [w448 _] -> w447
      tunnel: w445 -> [_ w449]
      event Timeout {
        n274 = event-data() -> ()  [unwired: 1 in, 3 out]
        n275 = local read "Stop All"() -> (w448:bool)
      }
      event "Record Diodes": Value Change {
        n276 = event-data() -> ()  [unwired: 1 in, 1 out]
        n277 = stacked-sequence {
          tunnel: w449 -> [_ w451 _]
          frame #0 {
            w450 = FALSE ("Record Diodes")
            "Record Diodes" <- w450
            "Diode read complete" <- w450
          }
          frame #1 {
            n278 = call "Build diode path.vi"("Data dir"=w451) -> ("Diode write path"=w452:path)  [unwired: 8 in, 1 out]
            n279 = call "Read Photodiodes.vi"("Diode tdms path"=w452) -> ()  [unwired: 3 in]
          }
          frame #2 {
            n280 = local write "Diode read complete"(TRUE ("Diode read complete")) -> ()
          }
        }
      }
    }
  }
  n281 = while {
    tunnel: w20 -> [w483]
    tunnel: w21 -> [w482]
    tunnel: [w474] -> w22
    tunnel: [w473] -> w23
    tunnel: w13 -> [_]
    tunnel: w7 -> [w460]
    stop <- w470 stop-if-true
    w463 = -114.181210191083  # intercept
    w466 = 1.11480891719745  # slope
    # "Pressure Read Loop"
    n282 = local read "Stop All"() -> (w470:bool)
    n283 = call "Read Pressure Transducers.vi"("Error In"=w482, "tdms file"=w460, "task in"=w483) -> ("Error Out"=w474:errorcluster, "Tube Pressure"=→"Tube Pressure":dbl[unit], "Manifold Pressure"=→"Manifold Pressure":dbl[unit], "task out"=w473:refnum<k21>, "Readings"=→"Pressure\nReadings":T3, "Calibration coefficients"=→"Pressure Calibration":T2)  [unwired: 3 in]
    n284 = local read "Manifold Pressure"() -> (w477:dbl[unit])
    n285 = local read "Oxidizer Cutoff"() -> (w480:dbl[unit])
    n286 = local read "Diluent Cutoff"() -> (w479:dbl[unit])
    n287 = local read "Tube Pressure"() -> (w469:dbl[unit])
    n288 = local read "Fuel Cutoff"() -> (w481:dbl[unit])
    n289 = local read "Atmospheric (Calibrated)"() -> (w456:dbl[unit])
    n290 = Bundle("Fuel Cutoff"=w481, "Oxidizer Cutoff"=w480, "Diluent Cutoff"=w479, "Manifold Pressure"=w477, "Tube Pressure"=w469) -> (→"System Pressures":T5)  [unwired: 1 in]
    n291 = node(w456) -> (w459:dbl)
    n292 = Greater Than 0?(x=w459) -> (x > 0?=w457:bool)
    n293 = Select(t=w456, s=w457, f=dbl[unit] 101325.0) -> (s? t:f=w455:dbl[unit])
    n294 = Multiply(x=1.25, y=w455) -> (x*y=w468:dbl[unit])
    n295 = Multiply(x="Atmospheric Pressure", y=w466) -> (x*y=w464:dbl[unit])
    n296 = Less?(x=w468, y=w469) -> (x < y?=→"Pressure Unsafe?":bool)
    n297 = node(w463) -> (w461:dbl[unit])
    n298 = Add(x=w464, y=w461) -> (x+y=→"Atmospheric (Calibrated)":dbl[unit])
  }
  n299 = while {
    tunnel: w14 -> [w487]
    tunnel: w15 -> [w486]
    stop <- w484 stop-if-true
    # "DAQ State Loop"
    n300 = event shown="[2] \"Current State\": Value Change" {
      selector: _ -> [_ _ _ _]
      dyn-events: _ -> [_ _ _ _]
      timeout: 100 -> [_ _ _ _]
      tunnel: w487 -> [_ w491 w510 _]
      tunnel: w486 -> [_ w490 w509 _]
      tunnel: [w488 w489 w508 _] -> w484
      event Timeout {
        n301 = event-data() -> ()  [unwired: 1 in, 3 out]
        n302 = local read "Stop Tests"() -> (w488:bool)
      }
      event "Valve Tube Outlet", "Valve Tube Inlet", "Valve Mix Outlet", "Valve Mix Inlet", "Mix Fan", "Valve Diluent", "Valve Fuel", "Valve Oxidizer", "Valve Purge", "Valve Vacuum", "Spark": Value Change {
        n303 = event-data() -> ()  [unwired: 1 in, 6 out]
        n304 = disable-structure shown="Default" {
          disable-tunnel: w491 -> [w496]
          disable-tunnel: w490 -> [w495]
          frame Enabled {
            # "Write instrument states to DAQ"
            n305 = local read "Valve Mix Outlet"() -> (w505:bool)
            n306 = disable-structure shown="Disabled" {
              frame Disabled {
                n307 = local read item#-1() -> ()  [unwired: 1 out]
              }
              frame Enabled {
              }
            }
            n308 = local read "Valve Tube Inlet"() -> (w507:bool)
            n309 = local read "Valve Purge"() -> (w500:bool)
            n310 = local read "Mix Fan"() -> (w497:bool)
            n311 = local read "Valve Fuel"() -> (w502:bool)
            n312 = local read "Valve Tube Outlet"() -> (w504:bool)
            n313 = local read "Valve Mix Inlet"() -> (w506:bool)
            n314 = local read "Valve Vacuum"() -> (w499:bool)
            n315 = local read "Valve Oxidizer"() -> (w503:bool)
            n316 = local read "Valve Diluent"() -> (w501:bool)
            n317 = local read "Spark"() -> (w498:bool)
            n318 = call "Read Tube Valves.vi"("task in"=w496, "Error In"=w495, "Tube Inlet"=w507, "Mix Inlet"=w506, "Mix Outlet"=w505, "Tube Outlet"=w504) -> ("Error Out"=w494:errorcluster)  [unwired: 8 in, 5 out]
            n319 = call "Read Manifold Valves.vi"("Task In"=w496, "Error In"=w494, "Oxidizer"=w503, "Fuel"=w502, "Diluent"=w501, "Purge"=w500, "Vacuum"=w499, "Manifold Outlet"=FALSE) -> ("Error Out"=w493:errorcluster)  [unwired: 12 in, 7 out]
            n320 = call "Instruments.vi"("task in"=w496, "Error In"=w493, "Spark"=w498, "Mix Fan"=w497) -> ()  [unwired: 12 in, 4 out]
          }
        }
        n321 = local read "Stop Tests"() -> (w489:bool)
      }
      event "Current State": Value Change {
        n322 = event-data() -> ()  [unwired: 1 in, 6 out]
        n323 = disable-structure shown="Default" {
          disable-tunnel: w510 -> [w526]
          disable-tunnel: w509 -> [w525]
          frame Enabled {
            n324 = case shown="\"Fuel Fill\"" "Current State" {
              tunnel: [FALSE ("Vacuum") FALSE ("Vacuum") FALSE ("Vacuum") FALSE ("Vacuum") TRUE ("Vacuum") FALSE ("Vacuum") FALSE ("Vacuum") FALSE ("Vacuum") FALSE ("Vacuum") FALSE ("Vacuum") FALSE ("Vacuum") FALSE ("Vacuum")] -> w517
              tunnel: [FALSE ("Manifold Outlet") FALSE ("Manifold Outlet") TRUE ("Manifold Outlet") FALSE ("Manifold Outlet") FALSE ("Manifold Outlet") FALSE ("Manifold Outlet") FALSE ("Manifold Outlet") FALSE ("Manifold Outlet") FALSE ("Manifold Outlet") FALSE ("Manifold Outlet") FALSE ("Manifold Outlet") FALSE ("Manifold Outlet")] -> w518
              tunnel: [FALSE ("Purge") FALSE ("Purge") FALSE ("Purge") TRUE ("Purge") FALSE ("Purge") FALSE ("Purge") FALSE ("Purge") FALSE ("Purge") FALSE ("Purge") FALSE ("Purge") FALSE ("Purge") FALSE ("Purge")] -> w519
              tunnel: [FALSE ("Oxidizer") FALSE ("Oxidizer") FALSE ("Oxidizer") FALSE ("Oxidizer") FALSE ("Oxidizer") FALSE ("Oxidizer") FALSE ("Oxidizer") FALSE ("Oxidizer") TRUE ("Oxidizer") TRUE ("Oxidizer") FALSE ("Oxidizer") FALSE ("Oxidizer")] -> w520
              tunnel: [FALSE ("Fuel") TRUE ("Fuel") FALSE ("Fuel") FALSE ("Fuel") FALSE ("Fuel") FALSE ("Fuel") FALSE ("Fuel") FALSE ("Fuel") FALSE ("Fuel") FALSE ("Fuel") FALSE ("Fuel") FALSE ("Fuel")] -> w516
              tunnel: [FALSE ("Diluent") TRUE ("Diluent") TRUE ("Diluent") TRUE ("Diluent") TRUE ("Diluent") FALSE ("Diluent") FALSE ("Diluent") FALSE ("Diluent") TRUE ("Diluent") TRUE ("Diluent") FALSE ("Diluent") FALSE ("Diluent")] -> _
              tunnel: [FALSE ("Tube Inlet") TRUE ("Tube Inlet") TRUE ("Tube Inlet") TRUE ("Tube Inlet") TRUE ("Tube Inlet") FALSE ("Tube Inlet") FALSE ("Tube Inlet") FALSE ("Tube Inlet") TRUE ("Tube Inlet") TRUE ("Tube Inlet") TRUE ("Tube Inlet") TRUE ("Tube Inlet")] -> w521
              tunnel: [TRUE ("Tube Outlet") FALSE ("Tube Outlet") FALSE ("Tube Outlet") FALSE ("Tube Outlet") FALSE ("Tube Outlet") FALSE ("Tube Outlet") FALSE ("Tube Outlet") FALSE ("Tube Outlet") TRUE ("Tube Outlet") TRUE ("Tube Outlet") FALSE ("Tube Outlet") TRUE ("Tube Outlet")] -> w524
              tunnel: [FALSE ("Mix Inlet") TRUE ("Mix Inlet") TRUE ("Mix Inlet") TRUE ("Mix Inlet") TRUE ("Mix Inlet") TRUE ("Mix Inlet") FALSE ("Mix Inlet") FALSE ("Mix Inlet") FALSE ("Mix Inlet") TRUE ("Mix Inlet") TRUE ("Mix Inlet") TRUE ("Mix Inlet")] -> w522
              tunnel: [FALSE ("Mix Outlet") TRUE ("Mix Outlet") TRUE ("Mix Outlet") TRUE ("Mix Outlet") TRUE ("Mix Outlet") TRUE ("Mix Outlet") FALSE ("Mix Outlet") FALSE ("Mix Outlet") FALSE ("Mix Outlet") TRUE ("Mix Outlet") TRUE ("Mix Outlet") TRUE ("Mix Outlet")] -> w523
              tunnel: [FALSE ("Oxidizer") FALSE ("Vacuum") FALSE ("Purge") FALSE ("Oxidizer") FALSE ("Purge") FALSE ("Oxidizer") FALSE ("Oxidizer") TRUE ("Oxidizer") FALSE ("Vacuum") FALSE ("Vacuum") FALSE ("Oxidizer") FALSE ("Oxidizer")] -> w515
              tunnel: [FALSE ("Fuel") FALSE ("Manifold Outlet") FALSE ("Oxidizer") FALSE ("Fuel") FALSE ("Oxidizer") TRUE ("Fuel") FALSE ("Fuel") FALSE ("Fuel") FALSE ("Manifold Outlet") TRUE ("Manifold Outlet") FALSE ("Fuel") FALSE ("Fuel")] -> w514
              tunnel: [FALSE ("Diluent") FALSE ("Purge") FALSE ("Fuel") FALSE ("Diluent") FALSE ("Fuel") FALSE ("Diluent") FALSE ("Diluent") FALSE ("Diluent") FALSE ("Purge") FALSE ("Purge") FALSE ("Diluent") FALSE ("Diluent")] -> w513
              frame "Tube Vent", Default {
              }
              frame "Tube Vacuum" {
              }
              frame "Fuel Fill" {
              }
              frame "Oxidizer Fill" {
              }
              frame "Diluent Fill" {
              }
              frame "Mixing" {
              }
              frame "Tube Closed" {
              }
              frame "Ignition" {
              }
              frame "Tube Purge" {
              }
              frame "Mix Section Purge" {
              }
              frame "Fill Hold" {
              }
              frame "Manifold Vent" {
              }
            }
            n325 = local write "Valve Oxidizer"(w519) -> ()
            n326 = local write "Valve Purge"(w520) -> ()
            n327 = local write "Valve Diluent"(w517) -> ()
            n328 = local write "Valve Fuel"(w518) -> ()
            n329 = local write "Valve Vacuum"(w516) -> ()
            n330 = local write "Valve Mix Inlet"(w522) -> ()
            n331 = local write "Valve Mix Outlet"(w523) -> ()
            n332 = local write "Valve Tube Inlet"(w521) -> ()
            n333 = local write "Valve Tube Outlet"(w524) -> ()
            n334 = local write "Mix Fan"(w514) -> ()
            n335 = local write "Spark"(w515) -> ()
            n336 = disable-structure shown="Default" {
              disable-tunnel: w521 -> [w541]
              disable-tunnel: w522 -> [w540]
              disable-tunnel: w523 -> [w539]
              disable-tunnel: w524 -> [w538]
              disable-tunnel: w517 -> [w537]
              disable-tunnel: w518 -> [w536]
              disable-tunnel: w520 -> [w535]
              disable-tunnel: w516 -> [w534]
              disable-tunnel: FALSE -> [w533]
              disable-tunnel: w515 -> [w532]
              disable-tunnel: w514 -> [w531]
              disable-tunnel: w513 -> [w530]
              disable-tunnel: w526 -> [w527]
              disable-tunnel: w525 -> [w529]
              disable-tunnel: w519 -> [w528]
              frame Enabled {
                # "Write instrument states to DAQ"
                n337 = call "Read Tube Valves.vi"("task in"=w527, "Error In"=w529, "Tube Inlet"=w541, "Mix Inlet"=w540, "Mix Outlet"=w539, "Tube Outlet"=w538) -> ("Error Out"=w543:errorcluster)  [unwired: 8 in, 5 out]
                n338 = call "Read Manifold Valves.vi"("Task In"=w527, "Error In"=w543, "Oxidizer"=w528, "Fuel"=w536, "Diluent"=w537, "Purge"=w535, "Vacuum"=w534, "Manifold Outlet"=w533) -> ("Error Out"=w542:errorcluster)  [unwired: 12 in, 7 out]
                n339 = call "Instruments.vi"("task in"=w527, "Error In"=w542, "Spark"=w532, "Mix Fan"=w531, "Camera"=w530) -> ()  [unwired: 11 in, 4 out]
              }
            }
          }
        }
        n340 = local read "Stop All"() -> (w508:bool)
      }
      event "Set Mode": Value Change {
        n341 = event-data() -> ()  [unwired: 1 in, 6 out]
        n342 = disable-structure shown="Default" {
          frame Enabled {
            # "Switch between test/run modes"
            n343 = Select(t=T6."Disabled" ("Disabled"), s="Set Mode", f=T6."Enabled" ("Disabled")) -> (s? t:f=w700:T6)
            n344 = property on="Valve Tube Inlet" class="Bool (strict)"("DisabledEnum"=w700) -> ()  [unwired: 2 in, 2 out]
            n345 = property on="Valve Mix Outlet" class="Bool (strict)"("DisabledEnum"=w700) -> ()  [unwired: 2 in, 2 out]
            n346 = property on="Valve Oxidizer" class="Bool (strict)"("DisabledEnum"=w700) -> ()  [unwired: 2 in, 2 out]
            n347 = property on="Valve Diluent" class="Bool (strict)"("DisabledEnum"=w700) -> ()  [unwired: 2 in, 2 out]
            n348 = property on="Valve Vacuum" class="Bool (strict)"("DisabledEnum"=w700) -> ()  [unwired: 2 in, 2 out]
            n349 = property on="Valve Fuel" class="Bool (strict)"("DisabledEnum"=w700) -> ()  [unwired: 2 in, 2 out]
            n350 = property on="Current State" class="Enum (strict)"("DisabledEnum"=w700) -> ()  [unwired: 2 in, 2 out]
            n351 = property on="Valve Tube Outlet" class="Bool (strict)"("DisabledEnum"=w700) -> ()  [unwired: 2 in, 2 out]
            n352 = property on="Valve Purge" class="Bool (strict)"("DisabledEnum"=w700) -> ()  [unwired: 2 in, 2 out]
            n353 = property on="Mix Fan" class="Bool (strict)"("DisabledEnum"=w700) -> ()  [unwired: 2 in, 2 out]
            n354 = property on="Valve Mix Inlet" class="Bool (strict)"("DisabledEnum"=w700) -> ()  [unwired: 2 in, 2 out]
          }
        }
      }
    }
  }
  n355 = call <vilib>:"DAQmx Clear Task.vi"("task in"=w18, "error in"=w19) -> ()  [unwired: 13 in, 1 out]
  n356 = event shown="[1] \"Stop Valve Control\": Value Change" {
    selector: _ -> [_ _]
    dyn-events: _ -> [_ _]
    timeout: _ -> [_ _]
    tunnel: w13 -> [_ w704]
    tunnel: [_ w704] -> w12
    event Timeout {
      n357 = event-data() -> ()  [unwired: 1 in, 3 out]
    }
    event "Stop Valve Control": Value Change {
      n358 = event-data() -> ()  [unwired: 1 in, 1 out]
      n359 = local write "Stop Tests"("Stop Valve Control") -> ()
    }
  }
  n360 = call <vilib>:"DAQmx Clear Task.vi"("task in"=w23, "error in"=w22) -> ()  [unwired: 13 in, 1 out]
  n361 = stacked-sequence "Shutdown sequence" {
    tunnel: w12 -> [_ _ _ _]
    tunnel: w7 -> [_ w710 _ _]
    tunnel: [_ w710 _ _] -> w6
    frame #0 {
      # "Vent until pressure is safe"
      n362 = property on="Current State" class="Enum (strict)"("Val(Sgnl)"=T4."Tube Vent" ("Value (Signaling)")) -> (error out=w706:errorcluster)  [unwired: 2 in, 1 out]
      n363 = while {
        tunnel: w706 -> [_]
        stop <- w708 stop-if-true
        # "Vent until pressure is safe"
        n364 = local read "Pressure Unsafe?"() -> (w709:bool)
        n365 = Not(x=w709) -> (.not. x?=w708:bool)
      }
    }
    frame #1 {
      # "Vent manifold"
      n366 = property on="Current State" class="Enum (strict)"("Val(Sgnl)"=T4."Manifold Vent" ("Value (Signaling)")) -> ()  [unwired: 2 in, 2 out]
      n367 = Wait (ms)(milliseconds to wait=u32 1000) -> ()  [unwired: 1 out]
    }
    frame #2 {
      # "Stop all loops"
      n368 = local write "Stop All"(TRUE ("Stop All")) -> ()
      n369 = Wait (ms)(milliseconds to wait=u32 1000) -> ()  [unwired: 1 out]
    }
    frame #3 {
      # "Reset DAQ"
      n370 = call <vilib>:"DAQmx Reset Device.vi"("device in"=tag "cDAQ1") -> ()  [unwired: 14 in, 1 out]
    }
  }
  n371 = TDMS Close(11:w6) -> ()  [unwired: 1 in, 2 out]
  "Test CSV" <- string[][] []
  "Test Status" <- "No tests loaded" ("Test Status")
  "Test CSV Header" <- w1
  "Test row" <- w1
